vi "Main.vi"() -> ()   [LabVIEW 2024]
uses:
  1. CTL/Brain_Loop_CTL.ctl
  <vilib>/Utility/miscctls.llb/LVPointTypeDef.ctl
  <vilib>/Utility/sysdir.llb/System Directory Type.ctl
panel:
  out "Water_Velocity 10":dbl
  out "Water_Velocity 9":dbl
  out "Water_Velocity 8":dbl
  out "Water_Velocity 7":dbl
  out "Water_Velocity 6":dbl
  out "Water_Velocity 5":dbl
  out "Water_Velocity 4":dbl
  out "Water_Velocity 3":dbl
  out "Water_Velocity 2":dbl
  out "Water_Velocity":dbl
  in  "숫자형":i32
  in  "유속 데이터 흐름표_50분":i32(listbox)=-1
  in  "유속 데이터 흐름표_30분":i32(listbox)=-1
  in  "유속 데이터 흐름표_10분":i32(listbox)=-1
  in  "유속 데이터":T1
  in  "데이터 통계":T2
  in  "관리자":T3
  out "반환값":string
  in  "전체메뉴_탭_컨트롤":enum32{"지도", "데이터 통계", "관리자", "유속 데이터"}(tab)=enum."데이터 통계"
  out "Station_5_수신시작시간":string
  out "Station_4_수신시작시간":string
  out "Station_3_수신시작시간":string
  out "Station_2_수신시작시간":string
  out "Station_1_수신시작시간":string
  out "Station_5":cluster{dbl[], i32[]}(graph)
  out "TX_LED_5":bool
  out "RX_LED_5":bool
  out "Station_4":cluster{dbl[], i32[]}(graph)
  out "TX_LED_4":bool
  out "RX_LED_4":bool
  out "Station_3":cluster{dbl[], i32[]}(graph)
  out "TX_LED_3":bool
  out "RX_LED_3":bool
  out "Station_2":cluster{dbl[], i32[]}(graph)
  out "TX_LED_2":bool
  out "RX_LED_2":bool
  out "Station_1":cluster{dbl[], i32[]}(graph)
  out "TX_LED_1":bool
  out "RX_LED_1":bool
  in  "관리자_내부_탭_컨트롤":enum32{"실시간 현황", "Setting"}(tab) caption="탭 컨트롤 2"
  out "Station_현황_GPS":i32[](listbox)
  out "데이터 통계 현황_결과창":string
  out "Station_현황_TRX_Controller":i32[](listbox)
  in  "Python 경로":path=path "D:/Python39-32/python.exe"
  out "적용_LED":bool
  in  "적용 버튼":bool
  in  "정지":bool
  in  "Publish_모듈 경로":path=path "C:/Users/user/Desktop/CATS_V4.0/5. Python/Mqtt_Publish_Client.py"
  in  "Subscribe_모듈 경로":path=path "C:/Users/user/Desktop/CATS_V4.0/5. Python/Mqtt_Subscribe_Client.py"
  in  "지도 모듈 경로":path=path "C:/Users/user/Desktop/CATS_V4.0/5. Python/Generate_map.py"
  out "적용_LED 2":bool
  in  "Wake_UP버튼":bool
  out "지도모듈_LED":bool
  in  "지도":T4
  in  "Order":i32=12
  in  "Q 값":i32=4
  # "Costal Acoustic Tomography(Ver1.1)"
  # "데이터 통계 현황"
  # "Costal Acoustic Tomography Setting"
  # "Data_path"
  # "Coastal_TMC_Set_Variable"
  # "Coastal_TMC_Map_Web"
  # "Sation_Wake_UP"
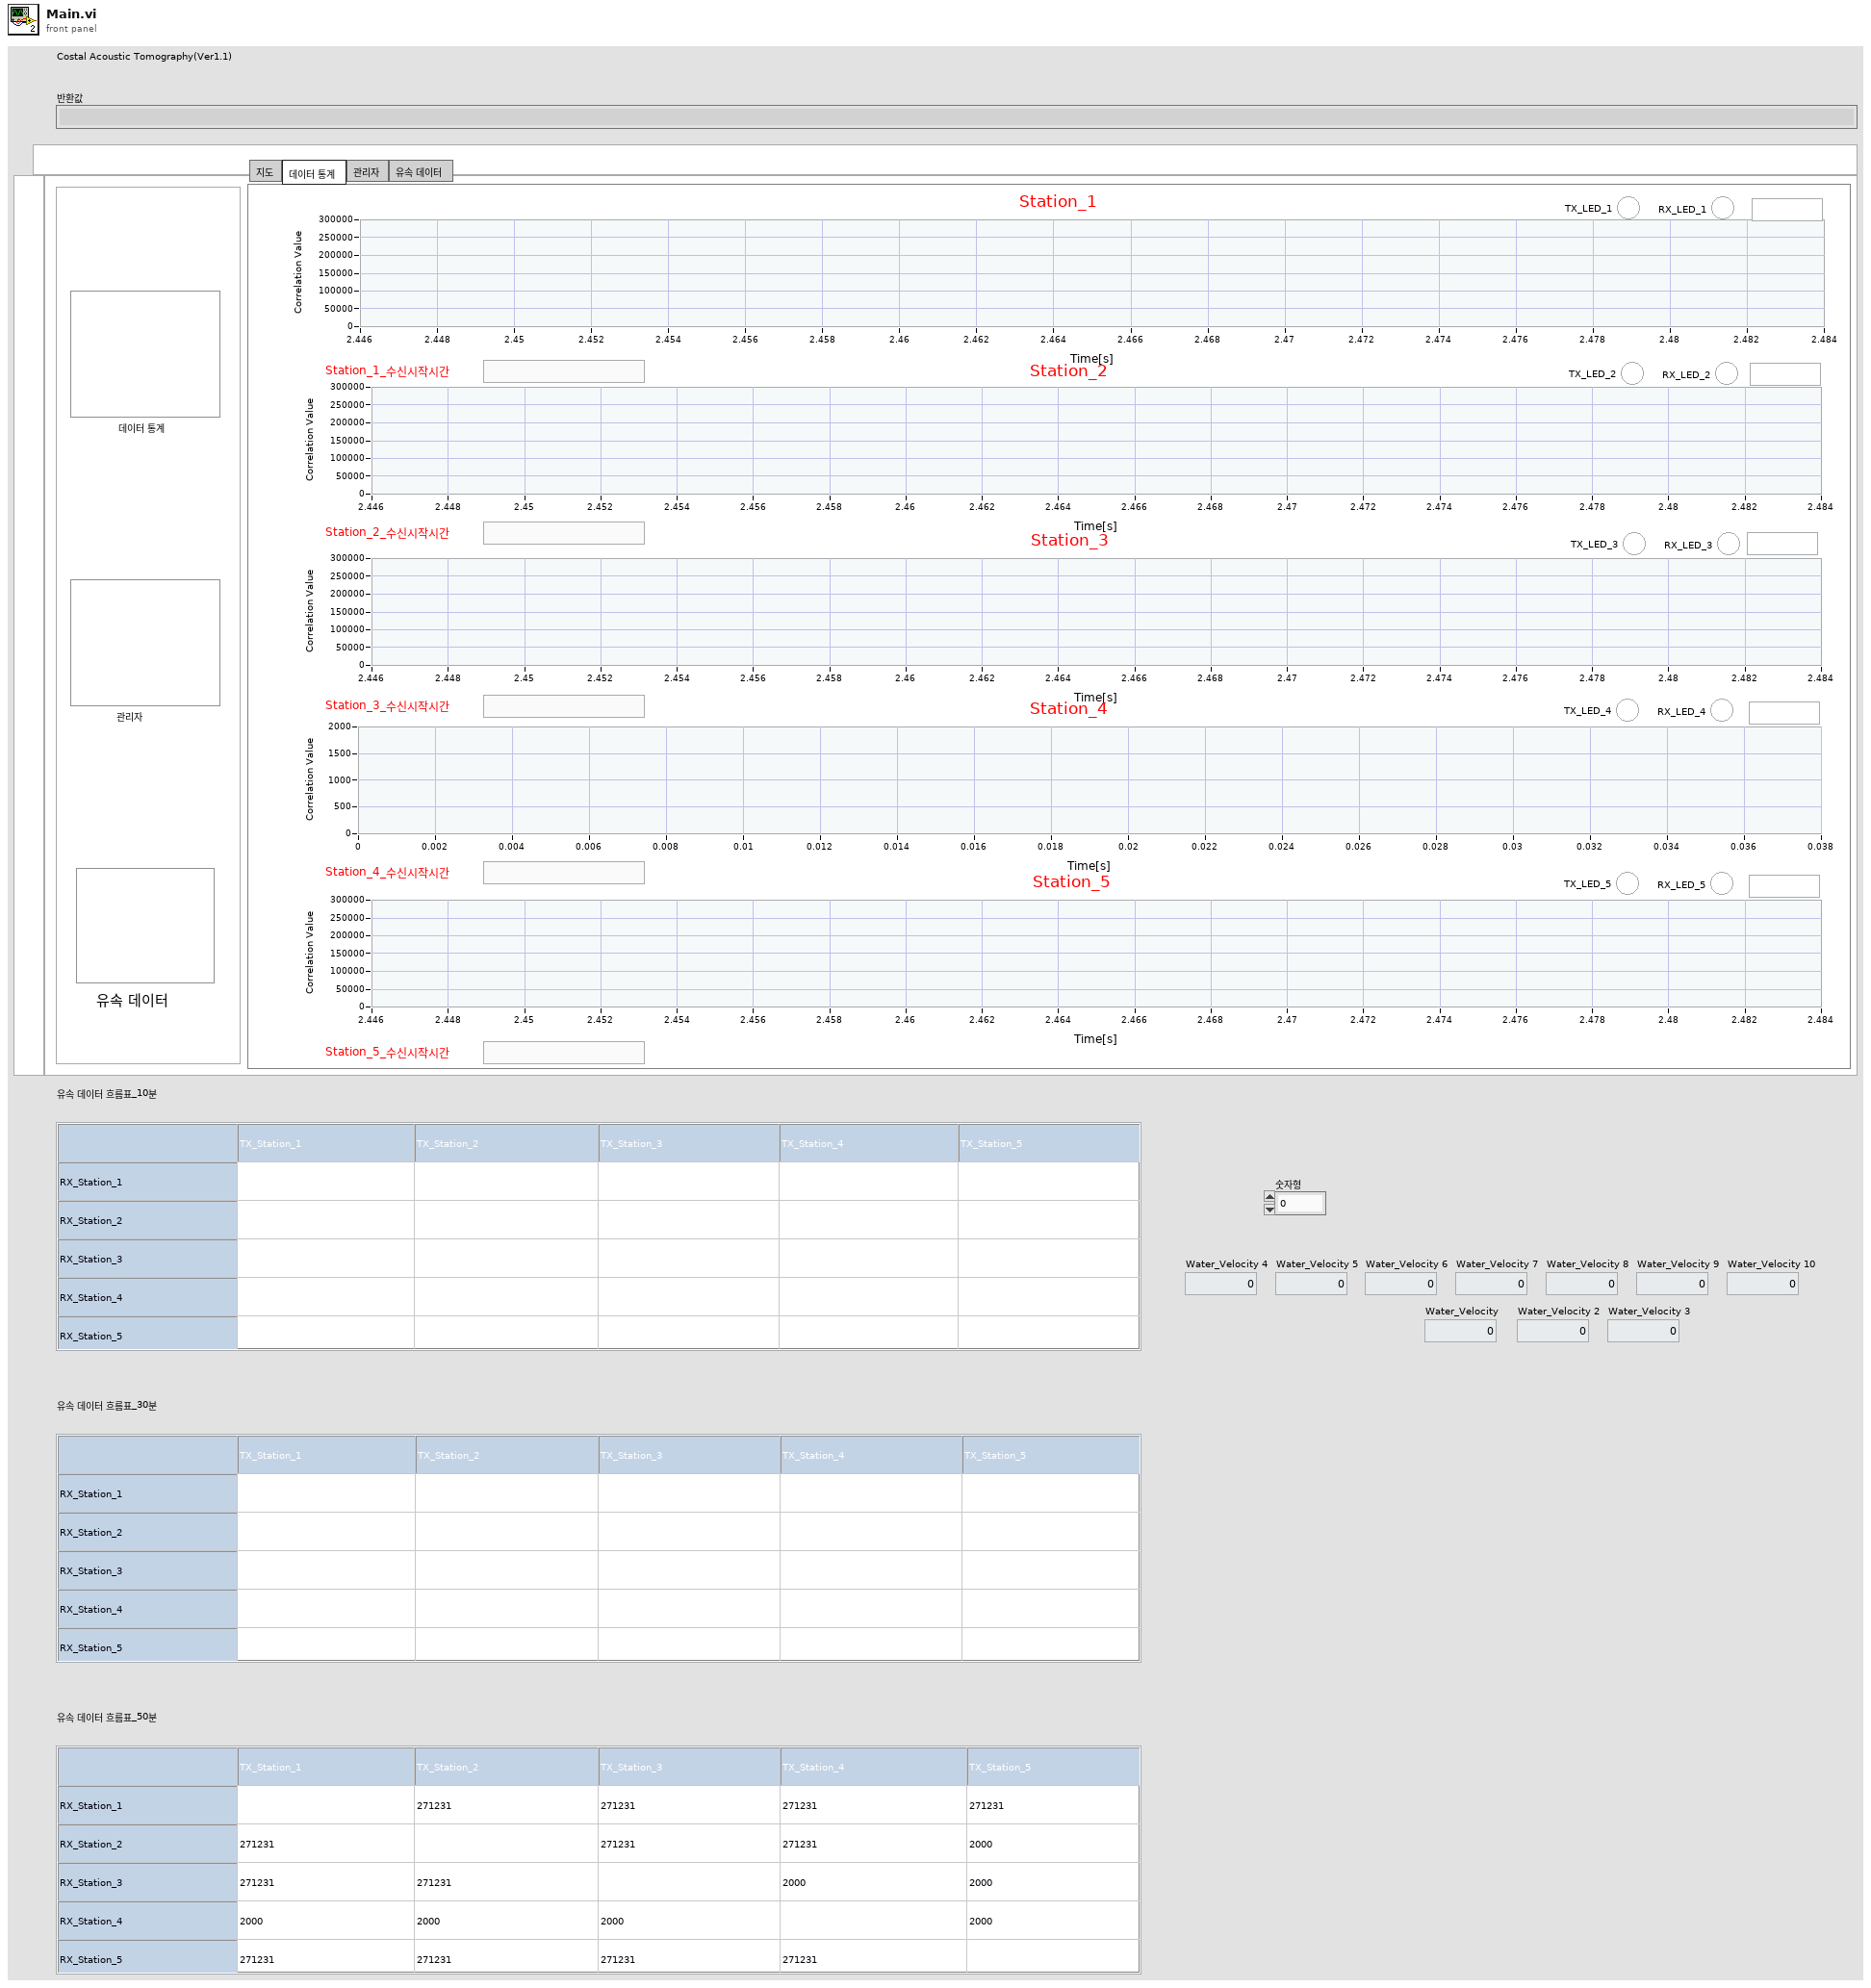
[diagram p1: front panel]
types:
  T1 = typedef "알림 컨트롤.ctl" = bool
  T2 = typedef "데이터 컨트롤.ctl" = bool
  T3 = typedef "관리 컨트롤.ctl" = bool
  T4 = typedef "지도 컨트롤.ctl" = bool
  T5 = cluster{"로그기록":string, "RX_그래프_LED":bool, "RX_그래프2_LED":bool, "RX_그래프3_LED":bool, "RX_그래프4_LED":bool, "RX_그래프5_LED":bool}
  T6 = cluster{"TX_그래프_LED":bool, "TX_그래프2_LED":bool, "TX_그래프3_LED":bool, "TX_그래프4_LED":bool, "TX_그래프5_LED":bool, "유속데이터흐름표_10분":string[][], "유속데이터흐름표_30분":string[][], "유속데이터흐름표_50분":string[][]}
  T7 = cluster{"Python 경로":path, "Publish 모듈 경로":path, "지도 모듈 경로":path}
  T8 = cluster{"TX_그래프_LED":bool, "TX_그래프2_LED":bool, "TX_그래프3_LED":bool, "TX_그래프4_LED":bool, "TX_그래프5_LED":bool}
  T9 = typedef "Brain_Loop_CTL.ctl" = enum16{"초기화", "Mqtt_Subscribe", "Mqtt_Publish", "지도", "관리자", "데이터통계", "유속 데이터", "정지", "Mqtt_Publish_2"}
  T10 = typedef "LVPointTypeDef.ctl" = cluster{"Horizontal":i16, "Vertical":i16}
  T11 = typedef "System Directory Type.ctl" = i32
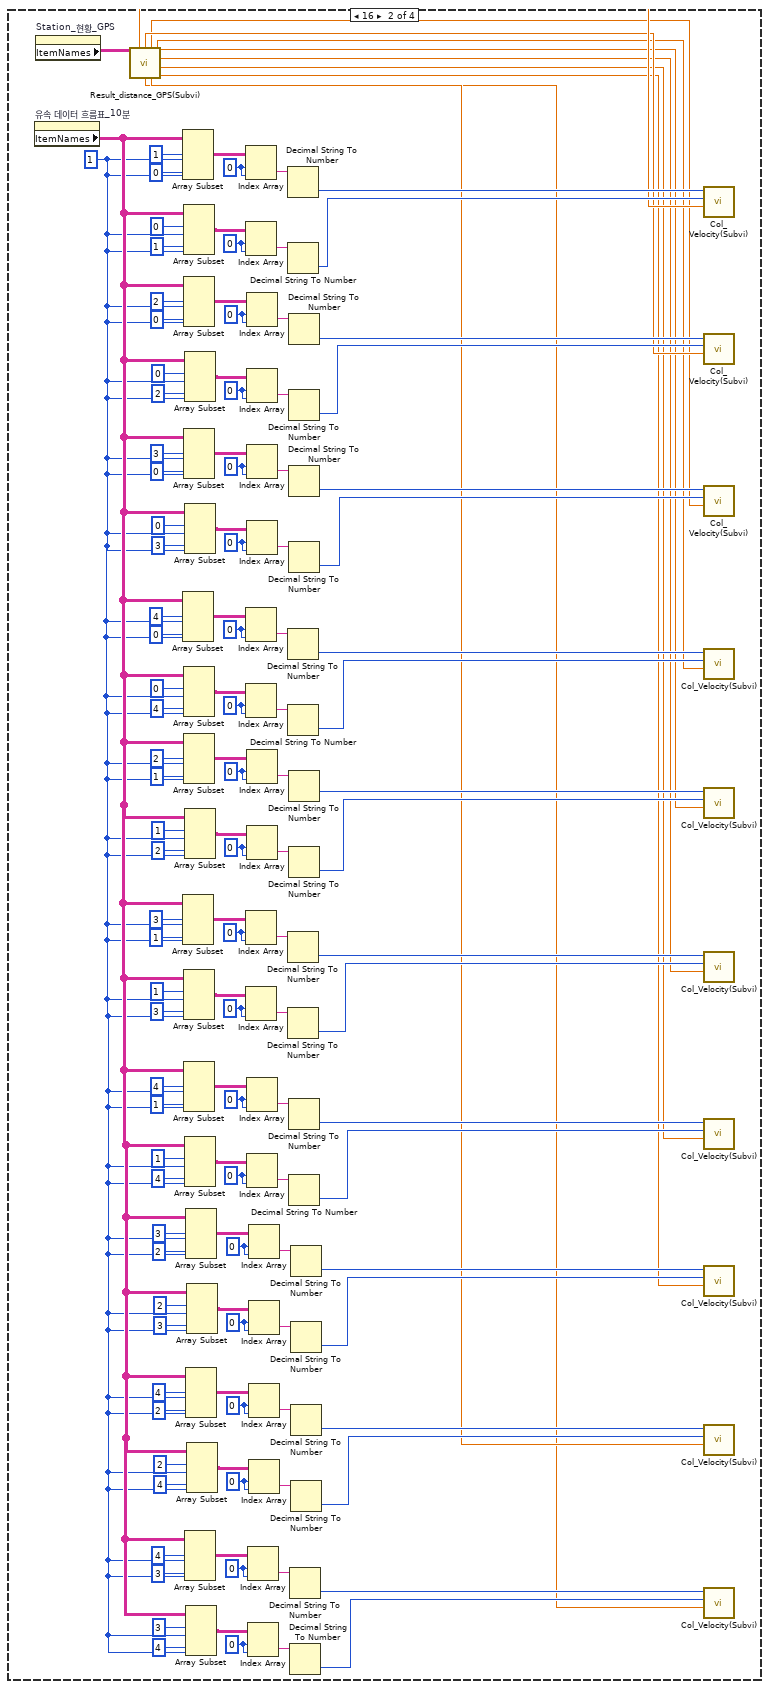
[diagram p3: hidden frame]
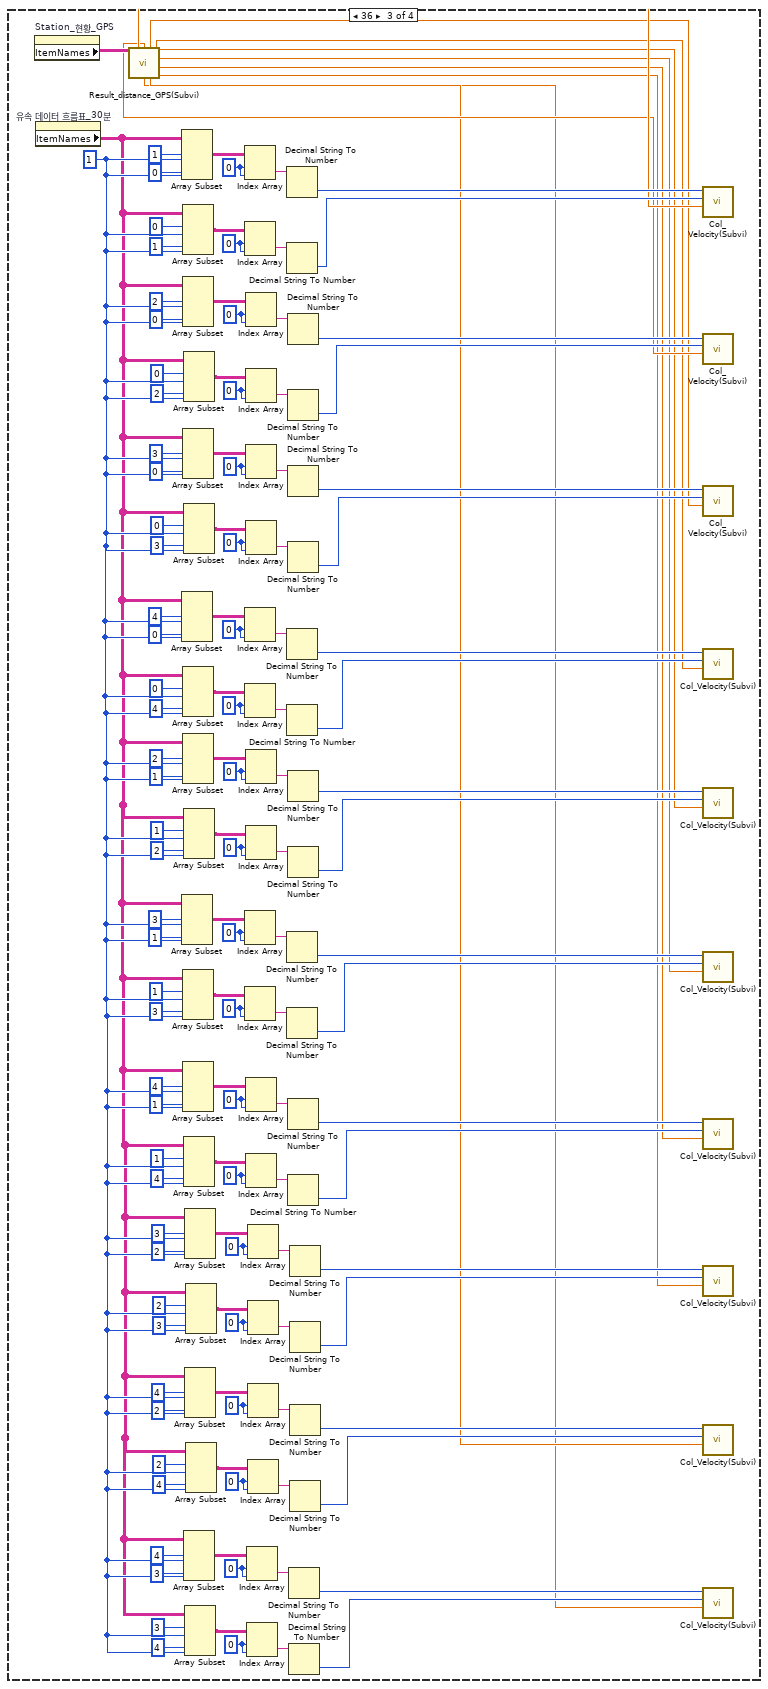
[diagram p4: hidden frame]
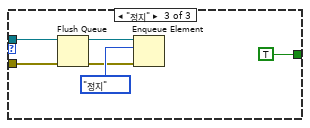
[diagram p6: hidden frame]
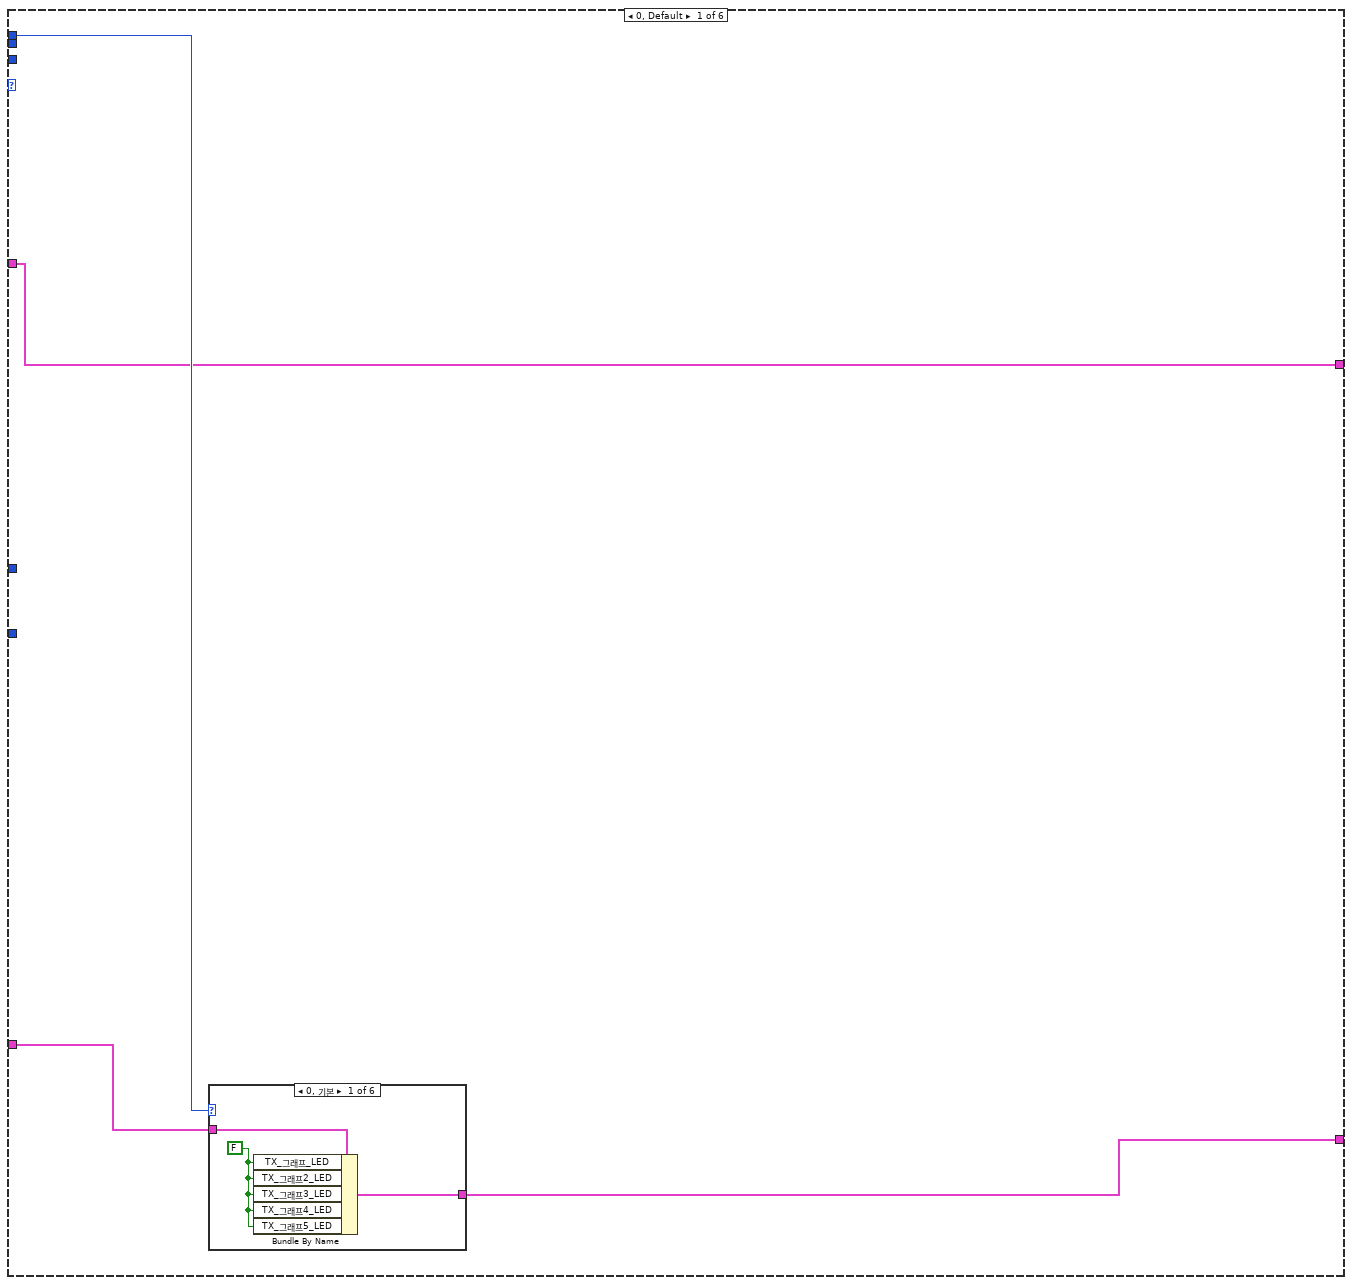
[diagram p7: hidden frame]
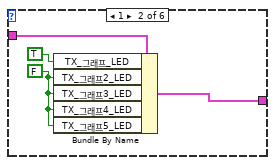
[diagram p8: hidden frame]
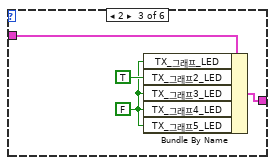
[diagram p9: hidden frame]
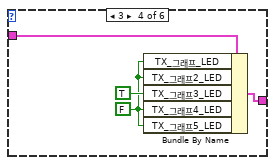
[diagram p10: hidden frame]
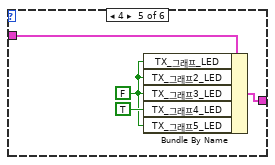
[diagram p11: hidden frame]
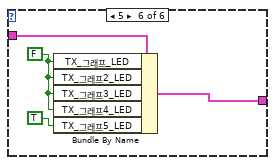
[diagram p12: hidden frame]
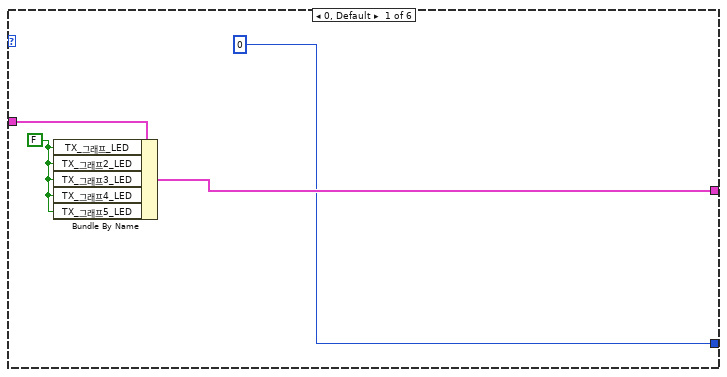
[diagram p13: hidden frame]
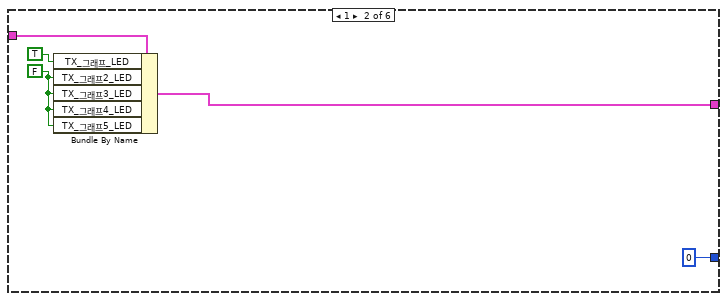
[diagram p14: hidden frame]
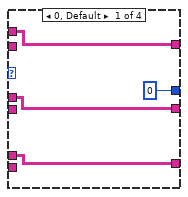
[diagram p15: hidden frame]
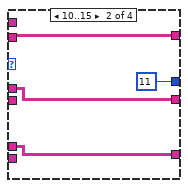
[diagram p16: hidden frame]
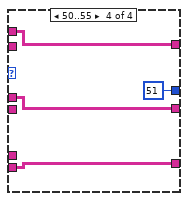
[diagram p17: hidden frame]
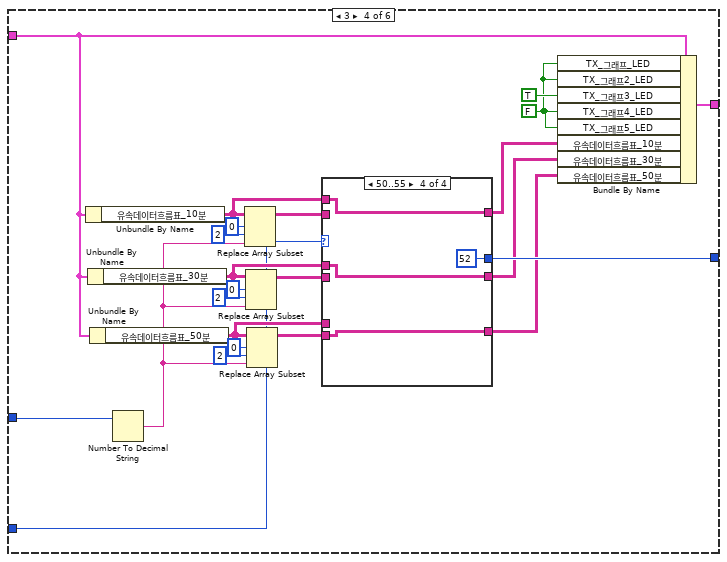
[diagram p18: hidden frame]
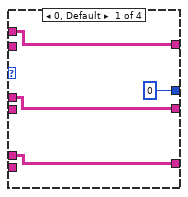
[diagram p19: hidden frame]
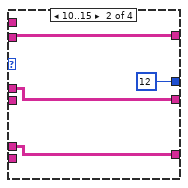
[diagram p20: hidden frame]
diagram:
  (unwired) T8 {"TX_그래프_LED"=FALSE, "TX_그래프2_LED"=FALSE, "TX_그래프3_LED"=FALSE, "TX_그래프4_LED"=FALSE, "TX_그래프5_LED"=FALSE}
  w20 = string[] []
  w21 = Brain_Loop_CTL."초기화"
  # "※ 현재 시간과 비교하여 10분 인지 30분인지 50분 출력 모듈 추가"
  # "Queue4: GPSDATA_처리 LOOP"
  # "GPS_리스트 박스 데이터 초기 값"
  # "TRX_Controller_리스트 박스 데이터 초기 값"
  # "Date: 2024.02.05\nTitle: Costal Acoustic Tmography GUI V1.1\nBy: KangJinSeong"
  n1 = Obtain Queue(element data type=w20) -> (queue out=w19:refnum<queue>, error out=w18:errorcluster)  [unwired: 4 in, 1 out]
  n2 = Obtain Queue(element data type=w20) -> (queue out=w7:refnum<queue>, error out=w6:errorcluster)  [unwired: 4 in, 1 out]
  n3 = Obtain Queue(element data type=w20) -> (queue out=w17:refnum<queue>, error out=w16:errorcluster)  [unwired: 4 in, 1 out]
  n4 = Obtain Queue(element data type=w21) -> (queue out=w24:refnum<queue>, error out=w26:errorcluster)  [unwired: 4 in, 1 out]
  n5 = Obtain Queue(element data type=w21) -> (queue out=w2:refnum<queue>, error out=w1:errorcluster)  [unwired: 4 in, 1 out]
  n6 = Enqueue Element(queue=w24, element=w21, error in (no error)=w26) -> (queue out=w15:refnum<queue>, error out=w25:errorcluster)  [unwired: 1 in, 1 out]
  n7 = while {
    tunnel: w15 -> [w29]
    shift-right: [w28] -> w23
    shift-left: w25 -> [w30]
    stop <- w27 stop-if-true
    n8 = event shown="[6] \"정지\": 값 변경" {
      selector: _ -> [_ _ _ _ _ _ _]
      dyn-events: _ -> [_ _ _ _ _ _ _]
      timeout: _ -> [_ _ _ _ _ _ _]
      tunnel: w30 -> [w35 w40 w42 w47 w55 w60 w66]
      tunnel: w29 -> [w34 w39 w44 w49 w54 w59 w65]
      tunnel: [w32 w37 w43 w48 w52 w58 w63] -> _
      tunnel: [w31 w36 w41 w46 w51 w57 w62] -> w28
      tunnel: [_ _ _ _ _ _ TRUE] -> w27
      event Value Change {
        n9 = event-data() -> ()  [unwired: 1 in, 1 out]
        n10 = Enqueue Element(queue=w34, element=Brain_Loop_CTL."지도", error in (no error)=w35) -> (queue out=w32:refnum<queue>, error out=w31:errorcluster)  [unwired: 1 in, 1 out]
      }
      event Value Change {
        n11 = event-data() -> ()  [unwired: 1 in, 1 out]
        n12 = Enqueue Element(queue=w39, element=Brain_Loop_CTL."데이터통계", error in (no error)=w40) -> (queue out=w37:refnum<queue>, error out=w36:errorcluster)  [unwired: 1 in, 1 out]
      }
      event "적용 버튼": Value Change {
        n13 = event-data() -> ()  [unwired: 1 in, 1 out]
        n14 = Enqueue Element(queue=w44, element=Brain_Loop_CTL."Mqtt_Publish", error in (no error)=w42) -> (queue out=w43:refnum<queue>, error out=w41:errorcluster)  [unwired: 1 in, 1 out]
      }
      event "Wake_UP버튼": Value Change {
        n15 = event-data() -> ()  [unwired: 1 in, 1 out]
        n16 = Enqueue Element(queue=w49, element=Brain_Loop_CTL."Mqtt_Publish_2", error in (no error)=w47) -> (queue out=w48:refnum<queue>, error out=w46:errorcluster)  [unwired: 1 in, 1 out]
      }
      event Value Change {
        n17 = event-data() -> ()  [unwired: 1 in, 1 out]
        n18 = Enqueue Element(queue=w54, element=Brain_Loop_CTL."관리자", error in (no error)=w55) -> (queue out=w52:refnum<queue>, error out=w51:errorcluster)  [unwired: 1 in, 1 out]
      }
      event Value Change {
        n19 = event-data() -> ()  [unwired: 1 in, 1 out]
        n20 = Enqueue Element(queue=w59, element=Brain_Loop_CTL."유속 데이터", error in (no error)=w60) -> (queue out=w58:refnum<queue>, error out=w57:errorcluster)  [unwired: 1 in, 1 out]
      }
      event "정지": Value Change {
        n21 = event-data() -> ()  [unwired: 1 in, 1 out]
        n22 = Enqueue Element(queue=w65, element=Brain_Loop_CTL."정지", error in (no error)=w66) -> (queue out=w63:refnum<queue>, error out=w62:errorcluster)  [unwired: 1 in, 1 out]
      }
    }
  }
  n23 = while {
    tunnel: w2 -> [w79]
    tunnel: w1 -> [w78]
    tunnel: w19 -> [w74]
    tunnel: w18 -> [w73]
    tunnel: [errorcluster {"status"=FALSE, "code"=0, "source"=""} ("에러 상수")] -> w12
    tunnel: w7 -> [w71]
    tunnel: w6 -> [w70]
    tunnel: w17 -> [w69]
    tunnel: w16 -> [w68]
    stop <- w77 stop-if-true
    # "Mqtt_Subscribe_Loop\n※ Brain_Loop의 Queue 값의 따라 작동(Mqtt_Subscribe, 정지, 초기화)"
    n24 = Dequeue Element(queue=w79, error in (no error)=w78) -> (queue out=w76:refnum<queue>, element=w67:T9, error out=w75:errorcluster)  [unwired: 1 in, 1 out]
    n25 = case shown="\"Mqtt_Subscribe\"" w67 {
      tunnel: [_ _ TRUE] -> w77
      tunnel: w76 -> [_ w100 w108]
      tunnel: w75 -> [_ w99 w107]
      tunnel: w74 -> [_ w97 _]
      tunnel: w73 -> [_ w96 _]
      tunnel: w71 -> [_ w95 _]
      tunnel: w70 -> [_ w94 _]
      tunnel: w69 -> [_ w93 _]
      tunnel: w68 -> [_ w92 _]
      frame "초기화", Default {
      }
      frame "Mqtt_Subscribe" {
        # "※ Queue 값의 따라 Python 모듈을 실행 해당 값을 통해 각 Loop 값에 데이터 전달"
        n26 = local read "Python 경로"() -> (w80:path)
        n27 = Enqueue Element(queue=w100, element=Brain_Loop_CTL."Mqtt_Subscribe", error in (no error)=w99) -> ()  [unwired: 1 in, 3 out]
        n28 = Open Python Session(python version="3.9" ("Python 버전"), python path=w80) -> (session out=w86:refnum<k35>, error out=w102:errorcluster)  [unwired: 1 in]
        n29 = node(w86, "Subscribe_모듈 경로", "Mqtt_Subscribe" ("함수 이름"), w102, "") -> (w88:refnum<k35>, w87:errorcluster, w83:string)  [unwired: 2 out]
        "반환값" <- w83
        n30 = Close Python Session(session in=w88, error in=w87) -> (11:w82:errorcluster)
        n31 = call "Split_Queue(Subvi).vi"("입력 문자열"=w83) -> ("Split_Queue2_Result"=w91:string[], "Split_Queue3_Result"=w90:string[], "Split_Queue4_Result"=w89:string[])  [unwired: 5 in, 3 out]
        n32 = call <vilib>:"Clear Errors.vi"("error in (no error)"=w82, "specific error code to clear (0: all)"=0) -> ()  [unwired: 4 in, 2 out]
        n33 = Enqueue Element(queue=w97, element=w91, error in (no error)=w96) -> ()  [unwired: 1 in, 3 out]
        n34 = Enqueue Element(queue=w93, element=w89, error in (no error)=w92) -> ()  [unwired: 1 in, 3 out]
        n35 = Enqueue Element(queue=w95, element=w90, error in (no error)=w94) -> ()  [unwired: 1 in, 3 out]
      }
      frame "정지" {
        # "※ Queue 값의 따라 정지 인경우 해당 큐를 비우고 정지 전달"
        n36 = Flush Queue(queue=w108, error in (no error)=w107) -> (queue out=w106:refnum<queue>, error out=w105:errorcluster)  [unwired: 1 out]
        n37 = Enqueue Element(queue=w106, element=Brain_Loop_CTL."정지", error in (no error)=w105) -> ()  [unwired: 1 in, 3 out]
      }
    }
  }
  n38 = while "While 루프" {
    tunnel: w2 -> [w144]
    tunnel: w1 -> [w143]
    tunnel: w7 -> [w142]
    tunnel: w6 -> [w141]
    shift-right: [w124] -> _
    shift-left: T6 {"TX_그래프_LED"=FALSE, "TX_그래프2_LED"=FALSE, "TX_그래프3_LED"=FALSE, "TX_그래프4_LED"=FALSE, "TX_그래프5_LED"=FALSE, "유속데이터흐름표_10분"=[["", "", "", "", "", ""], ["", "", "", "", "", ""], ["", "", "", "", "", ""], ["", "", "", "", "", ""], ["", "", "", "", "", ""], ["", "", "", "", "", "0"]], "유속데이터흐름표_30분"=[["", "", "", "", "", ""], ["", "", "", "", "", ""], ["", "", "", "", "", ""], ["", "", "", "", "", ""], ["", "", "", "", "", ""], ["", "", "", "", "", "0"]], "유속데이터흐름표_50분"=[["", "", "", "", "", ""], ["", "", "", "", "", ""], ["", "", "", "", "", ""], ["", "", "", "", "", ""], ["", "", "", "", "", ""], ["", "", "", "", "", "0"]]} -> [w130]
    shift-right: [w119] -> _
    shift-left: T5 {"로그기록"="", "RX_그래프_LED"=FALSE, "RX_그래프2_LED"=FALSE, "RX_그래프3_LED"=FALSE, "RX_그래프4_LED"=FALSE, "RX_그래프5_LED"=FALSE} -> [w123]
    stop <- w145 stop-if-true
    # "※ Queue3 처리 LOOP에 데이터가 들어오는 경우 각 인덱스에 맞게 데이터 분리 후 웨이브폼 그래프에 표시\n   TX_Station/RX_Station 값에 따라 .CSV 파일로 데이터 저장"
    # "※ TX_Station 번호 별로 그래프 하단에 LED 점멸(빨간색)\n    RX_Station 번호 별로 그래프 하단에 LED 점멸(파란색)"
    # "0 index: TX_Station\n1 index: RX_Station\n2 index: Max index"
    # "FPGA 신호처리된 결과값"
    # "Queue3: SIGDATA 처리 LOOP\n신호처리된 데이터 가시화 경우 시간 데이터로 표시"
    n39 = Dequeue Element(queue=w144, error in (no error)=w143) -> (queue out=w147:refnum<queue>, element=w146:T9, error out=w148:errorcluster)  [unwired: 1 in, 1 out]
    n40 = Dequeue Element(queue=w142, error in (no error)=w141) -> (element=w140:string[])  [unwired: 1 in, 3 out]
    n41 = case shown="\"Mqtt_Subscribe\"" w146 {
      tunnel: [_ _ TRUE] -> w145
      tunnel: w147 -> [_ w1327 w1332]
      tunnel: w148 -> [_ w1326 w1331]
      frame "초기화", Default {
      }
      frame "Mqtt_Subscribe" {
        n42 = Enqueue Element(queue=w1327, element=Brain_Loop_CTL."Mqtt_Subscribe", error in (no error)=w1326) -> ()  [unwired: 1 in, 3 out]
      }
      frame "정지" {
        n43 = Flush Queue(queue=w1332, error in (no error)=w1331) -> (queue out=w1330:refnum<queue>, error out=w1329:errorcluster)  [unwired: 1 out]
        n44 = Enqueue Element(queue=w1330, element=Brain_Loop_CTL."정지", error in (no error)=w1329) -> ()  [unwired: 1 in, 3 out]
      }
    }
    n45 = Decimal String To Number(string=w140) -> (number=w132:i32[])  [unwired: 2 in, 1 out]
    n46 = Array Subset(array=w132, index=4 ("인덱스"), length=4000 ("길이")) -> ()  [unwired: 1 out]
    n47 = Index Array(array=w132, index #1=1 ("인덱스"), index #2=0 ("인덱스"), index #3=2 ("인덱스")) -> (element #1=w133:i32, element #2=w134:i32, element #3=w131:i32)
    n48 = local read "Order"() -> (w121:i32)
    n49 = local read "Q 값"() -> (w122:i32)
    n50 = case shown="1" w133 {
      tunnel: w134 -> [w152 w209 w414 w642 w870 w1100]
      tunnel: w133 -> [_ w208 w435 w669 w898 w1128]
      tunnel: w132 -> [_ w225 w455 w685 w915 w1145]
      tunnel: w131 -> [_ w179 w411 w641 w869 w1099]
      tunnel: w130 -> [w151 w223 w413 w643 w871 w1101]
      tunnel: [w150 w222 w410 w639 w872 w1102] -> w124
      tunnel: w123 -> [w149 w205 w436 w670 w899 w1129]
      tunnel: w122 -> [_ w207 w438 w668 w897 w1127]
      tunnel: w121 -> [_ w206 w437 w667 w896 w1126]
      tunnel: [w149 w201 w439 w671 w900 w1130] -> w119
      tunnel: 50 -> [_ w176 w406 w636 w866 w1096]
      frame 0, Default {
        n51 = case shown="0, 기본" w152 {
          tunnel: w151 -> [w155 w159 w163 w167 w171 w175]
          tunnel: [w154 w156 w162 w166 w170 w174] -> w150
          frame 0, Default {
            w153 = FALSE
            n52 = Bundle By Name(cluster=w155, "TX_그래프_LED"=w153, "TX_그래프2_LED"=w153, "TX_그래프3_LED"=w153, "TX_그래프4_LED"=w153, "TX_그래프5_LED"=w153) -> (w154:T6)
          }
          frame 1 {
            w157 = FALSE
            n53 = Bundle By Name(cluster=w159, "TX_그래프_LED"=TRUE, "TX_그래프2_LED"=w157, "TX_그래프3_LED"=w157, "TX_그래프4_LED"=w157, "TX_그래프5_LED"=w157) -> (w156:T6)
          }
          frame 2 {
            w160 = FALSE
            n54 = Bundle By Name(cluster=w163, "TX_그래프_LED"=w160, "TX_그래프2_LED"=TRUE, "TX_그래프3_LED"=w160, "TX_그래프4_LED"=w160, "TX_그래프5_LED"=w160) -> (w162:T6)
          }
          frame 3 {
            w164 = FALSE
            n55 = Bundle By Name(cluster=w167, "TX_그래프_LED"=w164, "TX_그래프2_LED"=w164, "TX_그래프3_LED"=TRUE, "TX_그래프4_LED"=w164, "TX_그래프5_LED"=w164) -> (w166:T6)
          }
          frame 4 {
            w168 = FALSE
            n56 = Bundle By Name(cluster=w171, "TX_그래프_LED"=w168, "TX_그래프2_LED"=w168, "TX_그래프3_LED"=w168, "TX_그래프4_LED"=TRUE, "TX_그래프5_LED"=w168) -> (w170:T6)
          }
          frame 5 {
            w172 = FALSE
            n57 = Bundle By Name(cluster=w175, "TX_그래프_LED"=w172, "TX_그래프2_LED"=w172, "TX_그래프3_LED"=w172, "TX_그래프4_LED"=w172, "TX_그래프5_LED"=TRUE) -> (w174:T6)
          }
        }
      }
      frame 1 {
        w202 = FALSE
        # "※ 현재 시간과 비교하여 10분 인지 30분인지 50분 출력 모듈 추가"
        # "※2차원 벡터 -> 1차원 벡터"
        n58 = Subtract(x=w179, y=2000) -> (x-y=w228:i32)
        n59 = Format Date/Time String(time format string (%c)="%M" ("시간 포맷 문자열 (%c)")) -> (date/time string=w178:string)  [unwired: 2 in]
        n60 = call "Save_Log_File(Subvi).vi"("TX_Station"=w209, "RX_Station"=w208, "1D data"=w225) -> ()  [unwired: 7 in, 1 out]
        n61 = property on="Station_현황_TRX_Controller" class="MCListbox (엄격한)"() -> ("ItemNames"=w196:string[][])  [unwired: 2 in, 2 out]
        n62 = for {
          N: 4001 -> [_]
          tunnel: w228 -> [w405]
          shift-right: [w400] -> w226
          shift-left: dbl[] [] -> [w402]
          i -> [w399]
          n63 = Add(x=w405, y=w399) -> (x+y=w404:i32)
          n64 = Divide(x=w404, y=110000) -> (x/y=w401:dbl)
          n65 = Build Array (concatenate)(w402, w401) -> (w400:dbl[])
        }
        n66 = Unbundle By Name(w205) -> ("로그기록"=w210:string)
        n67 = Number To Decimal String(number=w209) -> (decimal integer string=w189:string)  [unwired: 1 in]
        n68 = Number To Decimal String(number=w208) -> (decimal integer string=w188:string)  [unwired: 1 in]
        n69 = Number To Decimal String(number=w179) -> (decimal integer string=w187:string)  [unwired: 1 in]
        n70 = Number To Decimal String(number=w207) -> (decimal integer string=w217:string)  [unwired: 1 in]
        n71 = Number To Decimal String(number=w206) -> (decimal integer string=w216:string)  [unwired: 1 in]
        n72 = Decimal String To Number(string=w178) -> ()  [unwired: 2 in, 2 out]
        n73 = Concatenate Strings("_Q_" ("시간 포맷 문자열 (%c)"), w217) -> (w214:string)
        n74 = Concatenate Strings("_Order : " ("시간 포맷 문자열 (%c)"), w216) -> (w213:string)
        n75 = case shown="2" w209 {
          tunnel: w223 -> [w237 w242 w256 w288 w327 w364]
          tunnel: [w236 w239 w259 w304 w343 w382] -> w222
          tunnel: [0 0 w263 w286 w325 w366] -> w199
          tunnel: w179 -> [_ _ w260 w287 w326 w365]
          tunnel: w176 -> [_ _ w243 w282 w321 w360]
          frame 0, Default {
            w235 = FALSE
            n76 = Bundle By Name(cluster=w237, "TX_그래프_LED"=w235, "TX_그래프2_LED"=w235, "TX_그래프3_LED"=w235, "TX_그래프4_LED"=w235, "TX_그래프5_LED"=w235) -> (w236:T6)
          }
          frame 1 {
            w240 = FALSE
            n77 = Bundle By Name(cluster=w242, "TX_그래프_LED"=TRUE, "TX_그래프2_LED"=w240, "TX_그래프3_LED"=w240, "TX_그래프4_LED"=w240, "TX_그래프5_LED"=w240) -> (w239:T6)
          }
          frame 2 {
            w264 = FALSE
            n78 = Unbundle By Name(w256) -> ("유속데이터흐름표_10분"=w244:string[][])
            n79 = Unbundle By Name(w256) -> ("유속데이터흐름표_30분"=w246:string[][])
            n80 = Unbundle By Name(w256) -> ("유속데이터흐름표_50분"=w245:string[][])
            n81 = Number To Decimal String(number=w260) -> (decimal integer string=w253:string)  [unwired: 1 in]
            n82 = Replace Array Subset(array=w244, new element=w253, index (row)=0 ("인덱스 (행)"), index (col)=1 ("비활성화된 인덱스 (열)")) -> (w252:string[][])
            n83 = Replace Array Subset(array=w246, new element=w253, index (row)=0 ("인덱스 (행)"), index (col)=1 ("비활성화된 인덱스 (열)")) -> (w251:string[][])
            n84 = Replace Array Subset(array=w245, new element=w253, index (row)=0 ("인덱스 (행)"), index (col)=1 ("비활성화된 인덱스 (열)")) -> (w250:string[][])
            n85 = case shown="30..35" w243 {
              tunnel: [0 11 31 51] -> w263
              tunnel: w252 -> [_ w272 _ _]
              tunnel: w251 -> [_ _ w275 _]
              tunnel: w250 -> [_ _ _ w278]
              tunnel: [w268 w272 w276 w280] -> w249
              tunnel: [w267 w271 w275 w279] -> w248
              tunnel: [w266 w270 w274 w278] -> w247
              tunnel: w246 -> [w267 w271 _ w279]
              tunnel: w245 -> [w266 w270 w274 _]
              tunnel: w244 -> [w268 _ w276 w280]
              frame 0, Default {
              }
              frame 10..15 {
              }
              frame 30..35 {
              }
              frame 50..55 {
              }
            }
            n86 = Bundle By Name(cluster=w256, "TX_그래프_LED"=w264, "TX_그래프2_LED"=TRUE, "TX_그래프3_LED"=w264, "TX_그래프4_LED"=w264, "TX_그래프5_LED"=w264, "유속데이터흐름표_10분"=w249, "유속데이터흐름표_30분"=w248, "유속데이터흐름표_50분"=w247) -> (w259:T6)
          }
          frame 3 {
            w302 = FALSE
            n87 = Unbundle By Name(w288) -> ("유속데이터흐름표_10분"=w301:string[][])
            n88 = Unbundle By Name(w288) -> ("유속데이터흐름표_30분"=w299:string[][])
            n89 = Unbundle By Name(w288) -> ("유속데이터흐름표_50분"=w300:string[][])
            n90 = Number To Decimal String(number=w287) -> (decimal integer string=w295:string)  [unwired: 1 in]
            n91 = Replace Array Subset(array=w301, new element=w295, index (row)=0 ("인덱스 (행)"), index (col)=2 ("비활성화된 인덱스 (열)")) -> (w296:string[][])
            n92 = Replace Array Subset(array=w299, new element=w295, index (row)=0 ("인덱스 (행)"), index (col)=2 ("비활성화된 인덱스 (열)")) -> (w297:string[][])
            n93 = Replace Array Subset(array=w300, new element=w295, index (row)=0 ("인덱스 (행)"), index (col)=2 ("비활성화된 인덱스 (열)")) -> (w298:string[][])
            n94 = case shown="50..55" w282 {
              tunnel: [0 12 32 52] -> w286
              tunnel: w296 -> [_ w311 _ _]
              tunnel: w297 -> [_ _ w314 _]
              tunnel: w298 -> [_ _ _ w317]
              tunnel: [w307 w311 w315 w319] -> w285
              tunnel: [w306 w310 w314 w318] -> w284
              tunnel: [w305 w309 w313 w317] -> w283
              tunnel: w299 -> [w306 w310 _ w318]
              tunnel: w300 -> [w305 w309 w313 _]
              tunnel: w301 -> [w307 _ w315 w319]
              frame 0, Default {
              }
              frame 10..15 {
              }
              frame 30..35 {
              }
              frame 50..55 {
              }
            }
            n95 = Bundle By Name(cluster=w288, "TX_그래프_LED"=w302, "TX_그래프2_LED"=w302, "TX_그래프3_LED"=TRUE, "TX_그래프4_LED"=w302, "TX_그래프5_LED"=w302, "유속데이터흐름표_10분"=w285, "유속데이터흐름표_30분"=w284, "유속데이터흐름표_50분"=w283) -> (w304:T6)
          }
          frame 4 {
            w341 = FALSE
            n96 = Unbundle By Name(w327) -> ("유속데이터흐름표_10분"=w340:string[][])
            n97 = Unbundle By Name(w327) -> ("유속데이터흐름표_30분"=w338:string[][])
            n98 = Unbundle By Name(w327) -> ("유속데이터흐름표_50분"=w339:string[][])
            n99 = Number To Decimal String(number=w326) -> (decimal integer string=w334:string)  [unwired: 1 in]
            n100 = Replace Array Subset(array=w340, new element=w334, index (row)=0 ("인덱스 (행)"), index (col)=3 ("비활성화된 인덱스 (열)")) -> (w335:string[][])
            n101 = Replace Array Subset(array=w338, new element=w334, index (row)=0 ("인덱스 (행)"), index (col)=3 ("비활성화된 인덱스 (열)")) -> (w336:string[][])
            n102 = Replace Array Subset(array=w339, new element=w334, index (row)=0 ("인덱스 (행)"), index (col)=3 ("비활성화된 인덱스 (열)")) -> (w337:string[][])
            n103 = case shown="10..15" w321 {
              tunnel: [0 13 33 53] -> w325
              tunnel: w335 -> [_ w350 _ _]
              tunnel: w336 -> [_ _ w353 _]
              tunnel: w337 -> [_ _ _ w356]
              tunnel: [w346 w350 w354 w358] -> w324
              tunnel: [w345 w349 w353 w357] -> w323
              tunnel: [w344 w348 w352 w356] -> w322
              tunnel: w338 -> [w345 w349 _ w357]
              tunnel: w339 -> [w344 w348 w352 _]
              tunnel: w340 -> [w346 _ w354 w358]
              frame 0, Default {
              }
              frame 10..15 {
              }
              frame 30..35 {
              }
              frame 50..55 {
              }
            }
            n104 = Bundle By Name(cluster=w327, "TX_그래프_LED"=w341, "TX_그래프2_LED"=w341, "TX_그래프3_LED"=w341, "TX_그래프4_LED"=TRUE, "TX_그래프5_LED"=w341, "유속데이터흐름표_10분"=w324, "유속데이터흐름표_30분"=w323, "유속데이터흐름표_50분"=w322) -> (w343:T6)
          }
          frame 5 {
            w380 = FALSE
            n105 = Unbundle By Name(w364) -> ("유속데이터흐름표_10분"=w379:string[][])
            n106 = Unbundle By Name(w364) -> ("유속데이터흐름표_30분"=w377:string[][])
            n107 = Unbundle By Name(w364) -> ("유속데이터흐름표_50분"=w378:string[][])
            n108 = Number To Decimal String(number=w365) -> (decimal integer string=w373:string)  [unwired: 1 in]
            n109 = Replace Array Subset(array=w379, new element=w373, index (row)=0 ("인덱스 (행)"), index (col)=4 ("비활성화된 인덱스 (열)")) -> (w374:string[][])
            n110 = Replace Array Subset(array=w377, new element=w373, index (row)=0 ("인덱스 (행)"), index (col)=4 ("비활성화된 인덱스 (열)")) -> (w375:string[][])
            n111 = Replace Array Subset(array=w378, new element=w373, index (row)=0 ("인덱스 (행)"), index (col)=4 ("비활성화된 인덱스 (열)")) -> (w376:string[][])
            n112 = case shown="50..55" w360 {
              tunnel: [0 14 34 54] -> w366
              tunnel: w374 -> [_ w389 _ _]
              tunnel: w375 -> [_ _ w392 _]
              tunnel: w376 -> [_ _ _ w395]
              tunnel: [w385 w389 w393 w397] -> w363
              tunnel: [w384 w388 w392 w396] -> w362
              tunnel: [w383 w387 w391 w395] -> w361
              tunnel: w377 -> [w384 w388 _ w396]
              tunnel: w378 -> [w383 w387 w391 _]
              tunnel: w379 -> [w385 _ w393 w397]
              frame 0, Default {
              }
              frame 10..15 {
              }
              frame 30..35 {
              }
              frame 50..55 {
              }
            }
            n113 = Bundle By Name(cluster=w364, "TX_그래프_LED"=w380, "TX_그래프2_LED"=w380, "TX_그래프3_LED"=w380, "TX_그래프4_LED"=w380, "TX_그래프5_LED"=TRUE, "유속데이터흐름표_10분"=w363, "유속데이터흐름표_30분"=w362, "유속데이터흐름표_50분"=w361) -> (w382:T6)
          }
        }
        n114 = Array Subset(array=w196, index (row)=0 ("인덱스"), length (row)=7 ("길이"), index (col)=0 ("인덱스"), length (col)=1 ("길이")) -> (w195:string[][])
        n115 = Format Date/Time String(time format string (%c)="%Y_%m_%d_%H_%M_" ("시간 포맷 문자열 (%c)")) -> (date/time string=w211:string)  [unwired: 2 in]
        n116 = Array Subset(array=w195, index (row)=3 ("인덱스"), length (row)=2 ("길이")) -> (w186:string[][])  [unwired: 2 in]
        n117 = Bundle(w226, w225) -> (→"Station_1":cluster{dbl[], i32[]})  [unwired: 1 in]
        n118 = for {
          tunnel: w186 -> [w232] mode=indexing
          shift-right: [w231] -> w184
          shift-left: string[] [] -> [w233]
          n119 = Build Array (concatenate)(w233, w232) -> (w231:string[])
        }
        n120 = Concatenate Strings(w210, w211, w189, "_Station_" ("시간 포맷 문자열 (%c)"), w188, "_Station : " ("시간 포맷 문자열 (%c)"), w187, w214, w213, "\r") -> (w204:string)
        n121 = Format Date/Time String(time format string (%c)="%Y_%m_%d_%H_" ("시간 포맷 문자열 (%c)")) -> (date/time string=w181:string)  [unwired: 2 in]
        n122 = Number To Decimal String(number=w199) -> (decimal integer string=w180:string)  [unwired: 1 in]
        n123 = Concatenate Strings(w181, w180) -> (→"Station_1_수신시작시간":string)
        n124 = Bundle By Name(cluster=w205, "로그기록"=w204, "RX_그래프_LED"=TRUE, "RX_그래프2_LED"=w202, "RX_그래프3_LED"=w202, "RX_그래프4_LED"=w202, "RX_그래프5_LED"=w202) -> (w201:T5)
        n125 = Build Array (concatenate)(w181, w180, w189, w188, w187, w184) -> (w183:string[])
        n126 = call "Save_teplete(Subvi).vi"("숫자형"=2, "배열"=w183) -> ()  [unwired: 10 in]
      }
      frame 2 {
        w409 = FALSE
        # "※ 2차원 벡터 -> 1차원 벡터"
        n127 = Subtract(x=w411, y=2000) -> (x-y=w458:i32)
        n128 = Format Date/Time String(time format string (%c)="%M" ("시간 포맷 문자열 (%c)")) -> (date/time string=w408:string)  [unwired: 2 in]
        n129 = call "Save_Log_File(Subvi).vi"("TX_Station"=w414, "RX_Station"=w435, "1D data"=w455) -> ()  [unwired: 7 in, 1 out]
        n130 = property on="Station_현황_TRX_Controller" class="MCListbox (엄격한)"() -> ("ItemNames"=w431:string[][])  [unwired: 2 in, 2 out]
        n131 = for {
          N: 4001 -> [_]
          tunnel: w458 -> [w635]
          shift-right: [w630] -> w456
          shift-left: dbl[] [] -> [w632]
          i -> [w629]
          n132 = Add(x=w635, y=w629) -> (x+y=w634:i32)
          n133 = Divide(x=w634, y=110000) -> (x/y=w631:dbl)
          n134 = Build Array (concatenate)(w632, w631) -> (w630:dbl[])
        }
        n135 = Decimal String To Number(string=w408) -> ()  [unwired: 2 in, 2 out]
        n136 = Unbundle By Name(w436) -> ("로그기록"=w442:string)
        n137 = Number To Decimal String(number=w414) -> (decimal integer string=w419:string)  [unwired: 1 in]
        n138 = Number To Decimal String(number=w435) -> (decimal integer string=w418:string)  [unwired: 1 in]
        n139 = Number To Decimal String(number=w411) -> (decimal integer string=w417:string)  [unwired: 1 in]
        n140 = Number To Decimal String(number=w438) -> (decimal integer string=w449:string)  [unwired: 1 in]
        n141 = Number To Decimal String(number=w437) -> (decimal integer string=w448:string)  [unwired: 1 in]
        n142 = case shown="5" w414 {
          tunnel: w413 -> [w464 w469 w505 w515 w554 w591]
          tunnel: [w463 w485 w506 w531 w570 w609] -> w410
          tunnel: [0 w471 0 w513 w552 w593] -> w412
          tunnel: w411 -> [_ w470 _ w514 w553 w592]
          tunnel: w406 -> [_ w465 _ w509 w548 w587]
          frame 0, Default {
            w462 = FALSE
            n143 = Bundle By Name(cluster=w464, "TX_그래프_LED"=w462, "TX_그래프2_LED"=w462, "TX_그래프3_LED"=w462, "TX_그래프4_LED"=w462, "TX_그래프5_LED"=w462) -> (w463:T6)
          }
          frame 1 {
            w486 = FALSE
            n144 = Unbundle By Name(w469) -> ("유속데이터흐름표_10분"=w472:string[][])
            n145 = Unbundle By Name(w469) -> ("유속데이터흐름표_30분"=w474:string[][])
            n146 = Unbundle By Name(w469) -> ("유속데이터흐름표_50분"=w473:string[][])
            n147 = Number To Decimal String(number=w470) -> (decimal integer string=w478:string)  [unwired: 1 in]
            n148 = Replace Array Subset(array=w472, new element=w478, index (row)=1 ("인덱스 (행)"), index (col)=0 ("비활성화된 인덱스 (열)")) -> (w477:string[][])
            n149 = Replace Array Subset(array=w474, new element=w478, index (row)=1 ("인덱스 (행)"), index (col)=0 ("비활성화된 인덱스 (열)")) -> (w476:string[][])
            n150 = Replace Array Subset(array=w473, new element=w478, index (row)=1 ("인덱스 (행)"), index (col)=0 ("비활성화된 인덱스 (열)")) -> (w475:string[][])
            n151 = case shown="0, 기본" w465 {
              tunnel: [0 10 30 50] -> w471
              tunnel: w477 -> [_ w494 _ _]
              tunnel: w476 -> [_ _ w497 _]
              tunnel: w475 -> [_ _ _ w500]
              tunnel: [w490 w494 w498 w502] -> w468
              tunnel: [w489 w493 w497 w501] -> w467
              tunnel: [w488 w492 w496 w500] -> w466
              tunnel: w474 -> [w489 w493 _ w501]
              tunnel: w473 -> [w488 w492 w496 _]
              tunnel: w472 -> [w490 _ w498 w502]
              frame 0, Default {
              }
              frame 10..15 {
              }
              frame 30..35 {
              }
              frame 50..55 {
              }
            }
            n152 = Bundle By Name(cluster=w469, "TX_그래프_LED"=TRUE, "TX_그래프2_LED"=w486, "TX_그래프3_LED"=w486, "TX_그래프4_LED"=w486, "TX_그래프5_LED"=w486, "유속데이터흐름표_10분"=w468, "유속데이터흐름표_30분"=w467, "유속데이터흐름표_50분"=w466) -> (w485:T6)
          }
          frame 2 {
            w507 = FALSE
            n153 = Bundle By Name(cluster=w505, "TX_그래프_LED"=w507, "TX_그래프2_LED"=TRUE, "TX_그래프3_LED"=w507, "TX_그래프4_LED"=w507, "TX_그래프5_LED"=w507) -> (w506:T6)
          }
          frame 3 {
            w529 = FALSE
            n154 = Unbundle By Name(w515) -> ("유속데이터흐름표_10분"=w528:string[][])
            n155 = Unbundle By Name(w515) -> ("유속데이터흐름표_30분"=w526:string[][])
            n156 = Unbundle By Name(w515) -> ("유속데이터흐름표_50분"=w527:string[][])
            n157 = Number To Decimal String(number=w514) -> (decimal integer string=w522:string)  [unwired: 1 in]
            n158 = Replace Array Subset(array=w528, new element=w522, index (row)=1 ("인덱스 (행)"), index (col)=2 ("비활성화된 인덱스 (열)")) -> (w523:string[][])
            n159 = Replace Array Subset(array=w526, new element=w522, index (row)=1 ("인덱스 (행)"), index (col)=2 ("비활성화된 인덱스 (열)")) -> (w524:string[][])
            n160 = Replace Array Subset(array=w527, new element=w522, index (row)=1 ("인덱스 (행)"), index (col)=2 ("비활성화된 인덱스 (열)")) -> (w525:string[][])
            n161 = case shown="50..55" w509 {
              tunnel: [0 12 32 52] -> w513
              tunnel: w523 -> [_ w538 _ _]
              tunnel: w524 -> [_ _ w541 _]
              tunnel: w525 -> [_ _ _ w544]
              tunnel: [w534 w538 w542 w546] -> w512
              tunnel: [w533 w537 w541 w545] -> w511
              tunnel: [w532 w536 w540 w544] -> w510
              tunnel: w526 -> [w533 w537 _ w545]
              tunnel: w527 -> [w532 w536 w540 _]
              tunnel: w528 -> [w534 _ w542 w546]
              frame 0, Default {
              }
              frame 10..15 {
              }
              frame 30..35 {
              }
              frame 50..55 {
              }
            }
            n162 = Bundle By Name(cluster=w515, "TX_그래프_LED"=w529, "TX_그래프2_LED"=w529, "TX_그래프3_LED"=TRUE, "TX_그래프4_LED"=w529, "TX_그래프5_LED"=w529, "유속데이터흐름표_10분"=w512, "유속데이터흐름표_30분"=w511, "유속데이터흐름표_50분"=w510) -> (w531:T6)
          }
          frame 4 {
            w568 = FALSE
            n163 = Unbundle By Name(w554) -> ("유속데이터흐름표_10분"=w567:string[][])
            n164 = Unbundle By Name(w554) -> ("유속데이터흐름표_30분"=w565:string[][])
            n165 = Unbundle By Name(w554) -> ("유속데이터흐름표_50분"=w566:string[][])
            n166 = Number To Decimal String(number=w553) -> (decimal integer string=w561:string)  [unwired: 1 in]
            n167 = Replace Array Subset(array=w567, new element=w561, index (row)=1 ("인덱스 (행)"), index (col)=3 ("비활성화된 인덱스 (열)")) -> (w562:string[][])
            n168 = Replace Array Subset(array=w565, new element=w561, index (row)=1 ("인덱스 (행)"), index (col)=3 ("비활성화된 인덱스 (열)")) -> (w563:string[][])
            n169 = Replace Array Subset(array=w566, new element=w561, index (row)=1 ("인덱스 (행)"), index (col)=3 ("비활성화된 인덱스 (열)")) -> (w564:string[][])
            n170 = case shown="10..15" w548 {
              tunnel: [0 13 33 53] -> w552
              tunnel: w562 -> [_ w577 _ _]
              tunnel: w563 -> [_ _ w580 _]
              tunnel: w564 -> [_ _ _ w583]
              tunnel: [w573 w577 w581 w585] -> w551
              tunnel: [w572 w576 w580 w584] -> w550
              tunnel: [w571 w575 w579 w583] -> w549
              tunnel: w565 -> [w572 w576 _ w584]
              tunnel: w566 -> [w571 w575 w579 _]
              tunnel: w567 -> [w573 _ w581 w585]
              frame 0, Default {
              }
              frame 10..15 {
              }
              frame 30..35 {
              }
              frame 50..55 {
              }
            }
            n171 = Bundle By Name(cluster=w554, "TX_그래프_LED"=w568, "TX_그래프2_LED"=w568, "TX_그래프3_LED"=w568, "TX_그래프4_LED"=TRUE, "TX_그래프5_LED"=w568, "유속데이터흐름표_10분"=w551, "유속데이터흐름표_30분"=w550, "유속데이터흐름표_50분"=w549) -> (w570:T6)
          }
          frame 5 {
            w607 = FALSE
            n172 = Unbundle By Name(w591) -> ("유속데이터흐름표_10분"=w606:string[][])
            n173 = Unbundle By Name(w591) -> ("유속데이터흐름표_30분"=w604:string[][])
            n174 = Unbundle By Name(w591) -> ("유속데이터흐름표_50분"=w605:string[][])
            n175 = Number To Decimal String(number=w592) -> (decimal integer string=w600:string)  [unwired: 1 in]
            n176 = Replace Array Subset(array=w606, new element=w600, index (row)=1 ("인덱스 (행)"), index (col)=4 ("비활성화된 인덱스 (열)")) -> (w601:string[][])
            n177 = Replace Array Subset(array=w604, new element=w600, index (row)=1 ("인덱스 (행)"), index (col)=4 ("비활성화된 인덱스 (열)")) -> (w602:string[][])
            n178 = Replace Array Subset(array=w605, new element=w600, index (row)=1 ("인덱스 (행)"), index (col)=4 ("비활성화된 인덱스 (열)")) -> (w603:string[][])
            n179 = case shown="0, 기본" w587 {
              tunnel: [0 14 34 54] -> w593
              tunnel: w601 -> [_ w616 _ _]
              tunnel: w602 -> [_ _ w619 _]
              tunnel: w603 -> [_ _ _ w622]
              tunnel: [w612 w616 w620 w624] -> w590
              tunnel: [w611 w615 w619 w623] -> w589
              tunnel: [w610 w614 w618 w622] -> w588
              tunnel: w604 -> [w611 w615 _ w623]
              tunnel: w605 -> [w610 w614 w618 _]
              tunnel: w606 -> [w612 _ w620 w624]
              frame 0, Default {
              }
              frame 10..15 {
              }
              frame 30..35 {
              }
              frame 50..55 {
              }
            }
            n180 = Bundle By Name(cluster=w591, "TX_그래프_LED"=w607, "TX_그래프2_LED"=w607, "TX_그래프3_LED"=w607, "TX_그래프4_LED"=w607, "TX_그래프5_LED"=TRUE, "유속데이터흐름표_10분"=w590, "유속데이터흐름표_30분"=w589, "유속데이터흐름표_50분"=w588) -> (w609:T6)
          }
        }
        n181 = Concatenate Strings("_Q_" ("시간 포맷 문자열 (%c)"), w449) -> (w446:string)
        n182 = Concatenate Strings("_Order : " ("시간 포맷 문자열 (%c)"), w448) -> (w445:string)
        n183 = Array Subset(array=w431, index (row)=0 ("인덱스"), length (row)=7 ("길이"), index (col)=0 ("인덱스"), length (col)=1 ("길이")) -> (w424:string[][])
        n184 = Format Date/Time String(time format string (%c)="%Y_%m_%d_%H_%M_" ("시간 포맷 문자열 (%c)")) -> (date/time string=w443:string)  [unwired: 2 in]
        n185 = Array Subset(array=w424, index (row)=3 ("인덱스"), length (row)=2 ("길이")) -> (w429:string[][])  [unwired: 2 in]
        n186 = Bundle(w456, w455) -> (→"Station_2":cluster{dbl[], i32[]})  [unwired: 1 in]
        n187 = for {
          tunnel: w429 -> [w627] mode=indexing
          shift-right: [w626] -> w416
          shift-left: string[] [] -> [w628]
          n188 = Build Array (concatenate)(w628, w627) -> (w626:string[])
        }
        n189 = Concatenate Strings(w442, w443, w419, "_Station_" ("시간 포맷 문자열 (%c)"), w418, "_Station : " ("시간 포맷 문자열 (%c)"), w417, w446, w445, "\r") -> (w441:string)
        n190 = Number To Decimal String(number=w412) -> (decimal integer string=w420:string)  [unwired: 1 in]
        n191 = Format Date/Time String(time format string (%c)="%Y_%m_%d_%H_" ("시간 포맷 문자열 (%c)")) -> (date/time string=w421:string)  [unwired: 2 in]
        n192 = Concatenate Strings(w421, w420) -> (→"Station_2_수신시작시간":string)
        n193 = Bundle By Name(cluster=w436, "로그기록"=w441, "RX_그래프_LED"=w409, "RX_그래프2_LED"=TRUE, "RX_그래프3_LED"=w409, "RX_그래프4_LED"=w409, "RX_그래프5_LED"=w409) -> (w439:T5)
        n194 = Build Array (concatenate)(w421, w420, w419, w418, w417, w416) -> (w415:string[])
        n195 = call "Save_teplete(Subvi).vi"("숫자형"=2, "배열"=w415) -> ()  [unwired: 10 in]
      }
      frame 3 {
        w665 = FALSE
        # "※2차원 벡터 -> 1차원 벡터"
        n196 = Format Date/Time String(time format string (%c)="%M" ("시간 포맷 문자열 (%c)")) -> (date/time string=w638:string)  [unwired: 2 in]
        n197 = Subtract(x=w641, y=2000) -> (x-y=w688:i32)
        n198 = call "Save_Log_File(Subvi).vi"("TX_Station"=w642, "RX_Station"=w669, "1D data"=w685) -> ()  [unwired: 7 in, 1 out]
        n199 = property on="Station_현황_TRX_Controller" class="MCListbox (엄격한)"() -> ("ItemNames"=w662:string[][])  [unwired: 2 in, 2 out]
        n200 = for {
          N: 4001 -> [_]
          tunnel: w688 -> [w865]
          shift-right: [w860] -> w686
          shift-left: dbl[] [] -> [w862]
          i -> [w859]
          n201 = Add(x=w865, y=w859) -> (x+y=w864:i32)
          n202 = Divide(x=w864, y=110000) -> (x/y=w861:dbl)
          n203 = Build Array (concatenate)(w862, w861) -> (w860:dbl[])
        }
        n204 = Decimal String To Number(string=w638) -> ()  [unwired: 2 in, 2 out]
        n205 = Unbundle By Name(w670) -> ("로그기록"=w673:string)
        n206 = Number To Decimal String(number=w642) -> (decimal integer string=w649:string)  [unwired: 1 in]
        n207 = Number To Decimal String(number=w669) -> (decimal integer string=w644:string)  [unwired: 1 in]
        n208 = Number To Decimal String(number=w641) -> (decimal integer string=w647:string)  [unwired: 1 in]
        n209 = Number To Decimal String(number=w668) -> (decimal integer string=w680:string)  [unwired: 1 in]
        n210 = Number To Decimal String(number=w667) -> (decimal integer string=w679:string)  [unwired: 1 in]
        n211 = case shown="5" w642 {
          tunnel: w643 -> [w694 w699 w739 w774 w784 w821]
          tunnel: [w693 w715 w754 w777 w800 w839] -> w639
          tunnel: [0 w701 w738 0 w782 w823] -> w640
          tunnel: w641 -> [_ w700 w740 _ w783 w822]
          tunnel: w636 -> [_ w695 w734 _ w778 w817]
          frame 0, Default {
            w692 = FALSE
            n212 = Bundle By Name(cluster=w694, "TX_그래프_LED"=w692, "TX_그래프2_LED"=w692, "TX_그래프3_LED"=w692, "TX_그래프4_LED"=w692, "TX_그래프5_LED"=w692) -> (w693:T6)
          }
          frame 1 {
            w716 = FALSE
            n213 = Unbundle By Name(w699) -> ("유속데이터흐름표_10분"=w702:string[][])
            n214 = Unbundle By Name(w699) -> ("유속데이터흐름표_30분"=w704:string[][])
            n215 = Unbundle By Name(w699) -> ("유속데이터흐름표_50분"=w703:string[][])
            n216 = Number To Decimal String(number=w700) -> (decimal integer string=w708:string)  [unwired: 1 in]
            n217 = Replace Array Subset(array=w702, new element=w708, index (row)=2 ("인덱스 (행)"), index (col)=0 ("비활성화된 인덱스 (열)")) -> (w707:string[][])
            n218 = Replace Array Subset(array=w704, new element=w708, index (row)=2 ("인덱스 (행)"), index (col)=0 ("비활성화된 인덱스 (열)")) -> (w706:string[][])
            n219 = Replace Array Subset(array=w703, new element=w708, index (row)=2 ("인덱스 (행)"), index (col)=0 ("비활성화된 인덱스 (열)")) -> (w705:string[][])
            n220 = case shown="10..15" w695 {
              tunnel: [0 10 30 50] -> w701
              tunnel: w707 -> [_ w724 _ _]
              tunnel: w706 -> [_ _ w727 _]
              tunnel: w705 -> [_ _ _ w730]
              tunnel: [w720 w724 w728 w732] -> w698
              tunnel: [w719 w723 w727 w731] -> w697
              tunnel: [w718 w722 w726 w730] -> w696
              tunnel: w704 -> [w719 w723 _ w731]
              tunnel: w703 -> [w718 w722 w726 _]
              tunnel: w702 -> [w720 _ w728 w732]
              frame 0, Default {
              }
              frame 10..15 {
              }
              frame 30..35 {
              }
              frame 50..55 {
              }
            }
            n221 = Bundle By Name(cluster=w699, "TX_그래프_LED"=TRUE, "TX_그래프2_LED"=w716, "TX_그래프3_LED"=w716, "TX_그래프4_LED"=w716, "TX_그래프5_LED"=w716, "유속데이터흐름표_10분"=w698, "유속데이터흐름표_30분"=w697, "유속데이터흐름표_50분"=w696) -> (w715:T6)
          }
          frame 2 {
            w755 = FALSE
            n222 = Unbundle By Name(w739) -> ("유속데이터흐름표_10분"=w741:string[][])
            n223 = Unbundle By Name(w739) -> ("유속데이터흐름표_30분"=w743:string[][])
            n224 = Unbundle By Name(w739) -> ("유속데이터흐름표_50분"=w742:string[][])
            n225 = Number To Decimal String(number=w740) -> (decimal integer string=w747:string)  [unwired: 1 in]
            n226 = Replace Array Subset(array=w741, new element=w747, index (row)=2 ("인덱스 (행)"), index (col)=1 ("비활성화된 인덱스 (열)")) -> (w746:string[][])
            n227 = Replace Array Subset(array=w743, new element=w747, index (row)=2 ("인덱스 (행)"), index (col)=1 ("비활성화된 인덱스 (열)")) -> (w745:string[][])
            n228 = Replace Array Subset(array=w742, new element=w747, index (row)=2 ("인덱스 (행)"), index (col)=1 ("비활성화된 인덱스 (열)")) -> (w744:string[][])
            n229 = case shown="50..55" w734 {
              tunnel: [0 11 31 51] -> w738
              tunnel: w746 -> [_ w763 _ _]
              tunnel: w745 -> [_ _ w766 _]
              tunnel: w744 -> [_ _ _ w769]
              tunnel: [w759 w763 w767 w771] -> w737
              tunnel: [w758 w762 w766 w770] -> w736
              tunnel: [w757 w761 w765 w769] -> w735
              tunnel: w743 -> [w758 w762 _ w770]
              tunnel: w742 -> [w757 w761 w765 _]
              tunnel: w741 -> [w759 _ w767 w771]
              frame 0, Default {
              }
              frame 10..15 {
              }
              frame 30..35 {
              }
              frame 50..55 {
              }
            }
            n230 = Bundle By Name(cluster=w739, "TX_그래프_LED"=w755, "TX_그래프2_LED"=TRUE, "TX_그래프3_LED"=w755, "TX_그래프4_LED"=w755, "TX_그래프5_LED"=w755, "유속데이터흐름표_10분"=w737, "유속데이터흐름표_30분"=w736, "유속데이터흐름표_50분"=w735) -> (w754:T6)
          }
          frame 3 {
            w775 = FALSE
            n231 = Bundle By Name(cluster=w774, "TX_그래프_LED"=w775, "TX_그래프2_LED"=w775, "TX_그래프3_LED"=TRUE, "TX_그래프4_LED"=w775, "TX_그래프5_LED"=w775) -> (w777:T6)
          }
          frame 4 {
            w798 = FALSE
            n232 = Unbundle By Name(w784) -> ("유속데이터흐름표_10분"=w797:string[][])
            n233 = Unbundle By Name(w784) -> ("유속데이터흐름표_30분"=w795:string[][])
            n234 = Unbundle By Name(w784) -> ("유속데이터흐름표_50분"=w796:string[][])
            n235 = Number To Decimal String(number=w783) -> (decimal integer string=w791:string)  [unwired: 1 in]
            n236 = Replace Array Subset(array=w797, new element=w791, index (row)=2 ("인덱스 (행)"), index (col)=3 ("비활성화된 인덱스 (열)")) -> (w792:string[][])
            n237 = Replace Array Subset(array=w795, new element=w791, index (row)=2 ("인덱스 (행)"), index (col)=3 ("비활성화된 인덱스 (열)")) -> (w793:string[][])
            n238 = Replace Array Subset(array=w796, new element=w791, index (row)=2 ("인덱스 (행)"), index (col)=3 ("비활성화된 인덱스 (열)")) -> (w794:string[][])
            n239 = case shown="10..15" w778 {
              tunnel: [0 13 33 53] -> w782
              tunnel: w792 -> [_ w807 _ _]
              tunnel: w793 -> [_ _ w810 _]
              tunnel: w794 -> [_ _ _ w813]
              tunnel: [w803 w807 w811 w815] -> w781
              tunnel: [w802 w806 w810 w814] -> w780
              tunnel: [w801 w805 w809 w813] -> w779
              tunnel: w795 -> [w802 w806 _ w814]
              tunnel: w796 -> [w801 w805 w809 _]
              tunnel: w797 -> [w803 _ w811 w815]
              frame 0, Default {
              }
              frame 10..15 {
              }
              frame 30..35 {
              }
              frame 50..55 {
              }
            }
            n240 = Bundle By Name(cluster=w784, "TX_그래프_LED"=w798, "TX_그래프2_LED"=w798, "TX_그래프3_LED"=w798, "TX_그래프4_LED"=TRUE, "TX_그래프5_LED"=w798, "유속데이터흐름표_10분"=w781, "유속데이터흐름표_30분"=w780, "유속데이터흐름표_50분"=w779) -> (w800:T6)
          }
          frame 5 {
            w837 = FALSE
            n241 = Unbundle By Name(w821) -> ("유속데이터흐름표_10분"=w836:string[][])
            n242 = Unbundle By Name(w821) -> ("유속데이터흐름표_30분"=w834:string[][])
            n243 = Unbundle By Name(w821) -> ("유속데이터흐름표_50분"=w835:string[][])
            n244 = Number To Decimal String(number=w822) -> (decimal integer string=w830:string)  [unwired: 1 in]
            n245 = Replace Array Subset(array=w836, new element=w830, index (row)=2 ("인덱스 (행)"), index (col)=4 ("비활성화된 인덱스 (열)")) -> (w831:string[][])
            n246 = Replace Array Subset(array=w834, new element=w830, index (row)=2 ("인덱스 (행)"), index (col)=4 ("비활성화된 인덱스 (열)")) -> (w832:string[][])
            n247 = Replace Array Subset(array=w835, new element=w830, index (row)=2 ("인덱스 (행)"), index (col)=4 ("비활성화된 인덱스 (열)")) -> (w833:string[][])
            n248 = case shown="10..15" w817 {
              tunnel: [0 14 34 54] -> w823
              tunnel: w831 -> [_ w846 _ _]
              tunnel: w832 -> [_ _ w849 _]
              tunnel: w833 -> [_ _ _ w852]
              tunnel: [w842 w846 w850 w854] -> w820
              tunnel: [w841 w845 w849 w853] -> w819
              tunnel: [w840 w844 w848 w852] -> w818
              tunnel: w834 -> [w841 w845 _ w853]
              tunnel: w835 -> [w840 w844 w848 _]
              tunnel: w836 -> [w842 _ w850 w854]
              frame 0, Default {
              }
              frame 10..15 {
              }
              frame 30..35 {
              }
              frame 50..55 {
              }
            }
            n249 = Bundle By Name(cluster=w821, "TX_그래프_LED"=w837, "TX_그래프2_LED"=w837, "TX_그래프3_LED"=w837, "TX_그래프4_LED"=w837, "TX_그래프5_LED"=TRUE, "유속데이터흐름표_10분"=w820, "유속데이터흐름표_30분"=w819, "유속데이터흐름표_50분"=w818) -> (w839:T6)
          }
        }
        n250 = Concatenate Strings("_Q_" ("시간 포맷 문자열 (%c)"), w680) -> (w677:string)
        n251 = Concatenate Strings("_Order : " ("시간 포맷 문자열 (%c)"), w679) -> (w676:string)
        n252 = Array Subset(array=w662, index (row)=0 ("인덱스"), length (row)=7 ("길이"), index (col)=0 ("인덱스"), length (col)=1 ("길이")) -> (w655:string[][])
        n253 = Format Date/Time String(time format string (%c)="%Y_%m_%d_%H_%M_" ("시간 포맷 문자열 (%c)")) -> (date/time string=w674:string)  [unwired: 2 in]
        n254 = Array Subset(array=w655, index (row)=3 ("인덱스"), length (row)=2 ("길이")) -> (w660:string[][])  [unwired: 2 in]
        n255 = Bundle(w686, w685) -> (→"Station_3":cluster{dbl[], i32[]})  [unwired: 1 in]
        n256 = for {
          tunnel: w660 -> [w857] mode=indexing
          shift-right: [w856] -> w646
          shift-left: string[] [] -> [w858]
          n257 = Build Array (concatenate)(w858, w857) -> (w856:string[])
        }
        n258 = Concatenate Strings(w673, w674, w649, "_Station_" ("시간 포맷 문자열 (%c)"), w644, "_Station : " ("시간 포맷 문자열 (%c)"), w647, w677, w676, "\r") -> (w672:string)
        n259 = Number To Decimal String(number=w640) -> (decimal integer string=w650:string)  [unwired: 1 in]
        n260 = Format Date/Time String(time format string (%c)="%Y_%m_%d_%H_" ("시간 포맷 문자열 (%c)")) -> (date/time string=w651:string)  [unwired: 2 in]
        n261 = Concatenate Strings(w651, w650) -> (→"Station_3_수신시작시간":string)
        n262 = Bundle By Name(cluster=w670, "로그기록"=w672, "RX_그래프_LED"=w665, "RX_그래프2_LED"=w665, "RX_그래프3_LED"=TRUE, "RX_그래프4_LED"=w665, "RX_그래프5_LED"=w665) -> (w671:T5)
        n263 = Build Array (concatenate)(w651, w650, w649, w644, w647, w646) -> (w645:string[])
        n264 = call "Save_teplete(Subvi).vi"("숫자형"=2, "배열"=w645) -> ()  [unwired: 10 in]
      }
      frame 4 {
        w894 = FALSE
        # "※2차원 벡터 -> 1차원 벡터"
        n265 = Format Date/Time String(time format string (%c)="%M" ("시간 포맷 문자열 (%c)")) -> (date/time string=w868:string)  [unwired: 2 in]
        n266 = Subtract(x=w869, y=2000) -> (x-y=w918:i32)
        n267 = Decimal String To Number(string=w868) -> ()  [unwired: 2 in, 2 out]
        n268 = call "Save_Log_File(Subvi).vi"("TX_Station"=w870, "RX_Station"=w898, "1D data"=w915) -> ()  [unwired: 7 in, 1 out]
        n269 = Unbundle By Name(w899) -> ("로그기록"=w902:string)
        n270 = Number To Decimal String(number=w870) -> (decimal integer string=w877:string)  [unwired: 1 in]
        n271 = Number To Decimal String(number=w898) -> (decimal integer string=w876:string)  [unwired: 1 in]
        n272 = Number To Decimal String(number=w869) -> (decimal integer string=w875:string)  [unwired: 1 in]
        n273 = Number To Decimal String(number=w897) -> (decimal integer string=w909:string)  [unwired: 1 in]
        n274 = Number To Decimal String(number=w896) -> (decimal integer string=w908:string)  [unwired: 1 in]
        n275 = for {
          N: 4001 -> [_]
          tunnel: w918 -> [w1095]
          shift-right: [w1090] -> w916
          shift-left: dbl[] [] -> [w1092]
          i -> [w1089]
          n276 = Add(x=w1095, y=w1089) -> (x+y=w1094:i32)
          n277 = Divide(x=w1094, y=110000) -> (x/y=w1091:dbl)
          n278 = Build Array (concatenate)(w1092, w1091) -> (w1090:dbl[])
        }
        n279 = case shown="1" w870 {
          tunnel: [w924 w945 w984 w1025 w1046 w1069] -> w872
          tunnel: [0 w934 w973 w1010 0 w1056] -> w873
          tunnel: w871 -> [w921 w930 w969 w1012 w1043 w1052]
          tunnel: w869 -> [_ w929 w968 w1011 _ w1051]
          tunnel: w866 -> [_ w925 w964 w1003 _ w1047]
          frame 0, Default {
            w923 = FALSE
            n280 = Bundle By Name(cluster=w921, "TX_그래프_LED"=w923, "TX_그래프2_LED"=w923, "TX_그래프3_LED"=w923, "TX_그래프4_LED"=w923, "TX_그래프5_LED"=w923) -> (w924:T6)
          }
          frame 1 {
            w946 = FALSE
            n281 = Unbundle By Name(w930) -> ("유속데이터흐름표_10분"=w928:string[][])
            n282 = Unbundle By Name(w930) -> ("유속데이터흐름표_30분"=w927:string[][])
            n283 = Unbundle By Name(w930) -> ("유속데이터흐름표_50분"=w926:string[][])
            n284 = Number To Decimal String(number=w929) -> (decimal integer string=w938:string)  [unwired: 1 in]
            n285 = Replace Array Subset(array=w928, new element=w938, index (row)=3 ("인덱스 (행)"), index (col)=0 ("비활성화된 인덱스 (열)")) -> (w937:string[][])
            n286 = Replace Array Subset(array=w927, new element=w938, index (row)=3 ("인덱스 (행)"), index (col)=0 ("비활성화된 인덱스 (열)")) -> (w936:string[][])
            n287 = Replace Array Subset(array=w926, new element=w938, index (row)=3 ("인덱스 (행)"), index (col)=0 ("비활성화된 인덱스 (열)")) -> (w935:string[][])
            n288 = case shown="50..55" w925 {
              tunnel: [0 10 30 50] -> w934
              tunnel: w937 -> [_ w954 _ _]
              tunnel: w936 -> [_ _ w958 _]
              tunnel: w935 -> [_ _ _ w962]
              tunnel: [w950 w954 w957 w961] -> w933
              tunnel: [w949 w953 w958 w960] -> w932
              tunnel: [w948 w952 w956 w962] -> w931
              tunnel: w927 -> [w949 w953 _ w960]
              tunnel: w926 -> [w948 w952 w956 _]
              tunnel: w928 -> [w950 _ w957 w961]
              frame 0, Default {
              }
              frame 10..15 {
              }
              frame 30..35 {
              }
              frame 50..55 {
              }
            }
            n289 = Bundle By Name(cluster=w930, "TX_그래프_LED"=TRUE, "TX_그래프2_LED"=w946, "TX_그래프3_LED"=w946, "TX_그래프4_LED"=w946, "TX_그래프5_LED"=w946, "유속데이터흐름표_10분"=w933, "유속데이터흐름표_30분"=w932, "유속데이터흐름표_50분"=w931) -> (w945:T6)
          }
          frame 2 {
            w985 = FALSE
            n290 = Unbundle By Name(w969) -> ("유속데이터흐름표_10분"=w967:string[][])
            n291 = Unbundle By Name(w969) -> ("유속데이터흐름표_30분"=w966:string[][])
            n292 = Unbundle By Name(w969) -> ("유속데이터흐름표_50분"=w965:string[][])
            n293 = Number To Decimal String(number=w968) -> (decimal integer string=w977:string)  [unwired: 1 in]
            n294 = Replace Array Subset(array=w967, new element=w977, index (row)=3 ("인덱스 (행)"), index (col)=1 ("비활성화된 인덱스 (열)")) -> (w976:string[][])
            n295 = Replace Array Subset(array=w966, new element=w977, index (row)=3 ("인덱스 (행)"), index (col)=1 ("비활성화된 인덱스 (열)")) -> (w975:string[][])
            n296 = Replace Array Subset(array=w965, new element=w977, index (row)=3 ("인덱스 (행)"), index (col)=1 ("비활성화된 인덱스 (열)")) -> (w974:string[][])
            n297 = case shown="10..15" w964 {
              tunnel: [0 11 31 51] -> w973
              tunnel: w976 -> [_ w993 _ _]
              tunnel: w975 -> [_ _ w997 _]
              tunnel: w974 -> [_ _ _ w1001]
              tunnel: [w989 w993 w996 w1000] -> w972
              tunnel: [w988 w992 w997 w999] -> w971
              tunnel: [w987 w991 w995 w1001] -> w970
              tunnel: w966 -> [w988 w992 _ w999]
              tunnel: w965 -> [w987 w991 w995 _]
              tunnel: w967 -> [w989 _ w996 w1000]
              frame 0, Default {
              }
              frame 10..15 {
              }
              frame 30..35 {
              }
              frame 50..55 {
              }
            }
            n298 = Bundle By Name(cluster=w969, "TX_그래프_LED"=w985, "TX_그래프2_LED"=TRUE, "TX_그래프3_LED"=w985, "TX_그래프4_LED"=w985, "TX_그래프5_LED"=w985, "유속데이터흐름표_10분"=w972, "유속데이터흐름표_30분"=w971, "유속데이터흐름표_50분"=w970) -> (w984:T6)
          }
          frame 3 {
            w1023 = FALSE
            n299 = Unbundle By Name(w1012) -> ("유속데이터흐름표_10분"=w1006:string[][])
            n300 = Unbundle By Name(w1012) -> ("유속데이터흐름표_30분"=w1005:string[][])
            n301 = Unbundle By Name(w1012) -> ("유속데이터흐름표_50분"=w1004:string[][])
            n302 = Number To Decimal String(number=w1011) -> (decimal integer string=w1016:string)  [unwired: 1 in]
            n303 = Replace Array Subset(array=w1006, new element=w1016, index (row)=3 ("인덱스 (행)"), index (col)=2 ("비활성화된 인덱스 (열)")) -> (w1015:string[][])
            n304 = Replace Array Subset(array=w1005, new element=w1016, index (row)=3 ("인덱스 (행)"), index (col)=2 ("비활성화된 인덱스 (열)")) -> (w1014:string[][])
            n305 = Replace Array Subset(array=w1004, new element=w1016, index (row)=3 ("인덱스 (행)"), index (col)=2 ("비활성화된 인덱스 (열)")) -> (w1013:string[][])
            n306 = case shown="10..15" w1003 {
              tunnel: [0 12 32 52] -> w1010
              tunnel: w1015 -> [_ w1032 _ _]
              tunnel: w1014 -> [_ _ w1036 _]
              tunnel: w1013 -> [_ _ _ w1040]
              tunnel: [w1028 w1032 w1035 w1039] -> w1009
              tunnel: [w1027 w1031 w1036 w1038] -> w1008
              tunnel: [w1026 w1030 w1034 w1040] -> w1007
              tunnel: w1005 -> [w1027 w1031 _ w1038]
              tunnel: w1004 -> [w1026 w1030 w1034 _]
              tunnel: w1006 -> [w1028 _ w1035 w1039]
              frame 0, Default {
              }
              frame 10..15 {
              }
              frame 30..35 {
              }
              frame 50..55 {
              }
            }
            n307 = Bundle By Name(cluster=w1012, "TX_그래프_LED"=w1023, "TX_그래프2_LED"=w1023, "TX_그래프3_LED"=TRUE, "TX_그래프4_LED"=w1023, "TX_그래프5_LED"=w1023, "유속데이터흐름표_10분"=w1009, "유속데이터흐름표_30분"=w1008, "유속데이터흐름표_50분"=w1007) -> (w1025:T6)
          }
          frame 4 {
            w1044 = FALSE
            n308 = Bundle By Name(cluster=w1043, "TX_그래프_LED"=w1044, "TX_그래프2_LED"=w1044, "TX_그래프3_LED"=w1044, "TX_그래프4_LED"=TRUE, "TX_그래프5_LED"=w1044) -> (w1046:T6)
          }
          frame 5 {
            w1067 = FALSE
            n309 = Unbundle By Name(w1052) -> ("유속데이터흐름표_10분"=w1050:string[][])
            n310 = Unbundle By Name(w1052) -> ("유속데이터흐름표_30분"=w1049:string[][])
            n311 = Unbundle By Name(w1052) -> ("유속데이터흐름표_50분"=w1048:string[][])
            n312 = Number To Decimal String(number=w1051) -> (decimal integer string=w1063:string)  [unwired: 1 in]
            n313 = Replace Array Subset(array=w1050, new element=w1063, index (row)=3 ("인덱스 (행)"), index (col)=4 ("비활성화된 인덱스 (열)")) -> (w1064:string[][])
            n314 = Replace Array Subset(array=w1049, new element=w1063, index (row)=3 ("인덱스 (행)"), index (col)=4 ("비활성화된 인덱스 (열)")) -> (w1065:string[][])
            n315 = Replace Array Subset(array=w1048, new element=w1063, index (row)=3 ("인덱스 (행)"), index (col)=4 ("비활성화된 인덱스 (열)")) -> (w1066:string[][])
            n316 = case shown="10..15" w1047 {
              tunnel: [0 14 34 54] -> w1056
              tunnel: w1064 -> [_ w1076 _ _]
              tunnel: w1065 -> [_ _ w1080 _]
              tunnel: w1066 -> [_ _ _ w1084]
              tunnel: [w1072 w1076 w1079 w1083] -> w1055
              tunnel: [w1071 w1075 w1080 w1082] -> w1054
              tunnel: [w1070 w1074 w1078 w1084] -> w1053
              tunnel: w1049 -> [w1071 w1075 _ w1082]
              tunnel: w1048 -> [w1070 w1074 w1078 _]
              tunnel: w1050 -> [w1072 _ w1079 w1083]
              frame 0, Default {
              }
              frame 10..15 {
              }
              frame 30..35 {
              }
              frame 50..55 {
              }
            }
            n317 = Bundle By Name(cluster=w1052, "TX_그래프_LED"=w1067, "TX_그래프2_LED"=w1067, "TX_그래프3_LED"=w1067, "TX_그래프4_LED"=w1067, "TX_그래프5_LED"=TRUE, "유속데이터흐름표_10분"=w1055, "유속데이터흐름표_30분"=w1054, "유속데이터흐름표_50분"=w1053) -> (w1069:T6)
          }
        }
        n318 = Concatenate Strings("_Q_" ("시간 포맷 문자열 (%c)"), w909) -> (w906:string)
        n319 = Concatenate Strings("_Order : " ("시간 포맷 문자열 (%c)"), w908) -> (w905:string)
        n320 = Format Date/Time String(time format string (%c)="%Y_%m_%d_%H_%M_" ("시간 포맷 문자열 (%c)")) -> (date/time string=w903:string)  [unwired: 2 in]
        n321 = Bundle(w916, w915) -> (→"Station_4":cluster{dbl[], i32[]})  [unwired: 1 in]
        n322 = Concatenate Strings(w902, w903, w877, "_Station_" ("시간 포맷 문자열 (%c)"), w876, "_Station : " ("시간 포맷 문자열 (%c)"), w875, w906, w905, "\r") -> (w901:string)
        n323 = property on="Station_현황_TRX_Controller" class="MCListbox (엄격한)"() -> ("ItemNames"=w891:string[][])  [unwired: 2 in, 2 out]
        n324 = Array Subset(array=w891, index (row)=0 ("인덱스"), length (row)=7 ("길이"), index (col)=0 ("인덱스"), length (col)=1 ("길이")) -> (w884:string[][])
        n325 = Array Subset(array=w884, index (row)=3 ("인덱스"), length (row)=2 ("길이")) -> (w889:string[][])  [unwired: 2 in]
        n326 = for {
          tunnel: w889 -> [w1087] mode=indexing
          shift-right: [w1086] -> w874
          shift-left: string[] [] -> [w1088]
          n327 = Build Array (concatenate)(w1088, w1087) -> (w1086:string[])
        }
        n328 = Format Date/Time String(time format string (%c)="%Y_%m_%d_%H_" ("시간 포맷 문자열 (%c)")) -> (date/time string=w880:string)  [unwired: 2 in]
        n329 = Number To Decimal String(number=w873) -> (decimal integer string=w879:string)  [unwired: 1 in]
        n330 = Concatenate Strings(w880, w879) -> (→"Station_4_수신시작시간":string)
        n331 = Bundle By Name(cluster=w899, "로그기록"=w901, "RX_그래프_LED"=w894, "RX_그래프2_LED"=w894, "RX_그래프3_LED"=w894, "RX_그래프4_LED"=TRUE, "RX_그래프5_LED"=w894) -> (w900:T5)
        n332 = Build Array (concatenate)(w880, w879, w877, w876, w875, w874) -> (w878:string[])
        n333 = call "Save_teplete(Subvi).vi"("숫자형"=2, "배열"=w878) -> ()  [unwired: 10 in]
      }
      frame 5 {
        w1124 = FALSE
        # "※2차원 벡터 -> 1차원 벡터"
        n334 = Format Date/Time String(time format string (%c)="%M" ("시간 포맷 문자열 (%c)")) -> (date/time string=w1098:string)  [unwired: 2 in]
        n335 = property on="Station_현황_TRX_Controller" class="MCListbox (엄격한)"() -> ("ItemNames"=w1121:string[][])  [unwired: 2 in, 2 out]
        n336 = Subtract(x=w1099, y=2000) -> (x-y=w1148:i32)
        n337 = Decimal String To Number(string=w1098) -> ()  [unwired: 2 in, 2 out]
        n338 = call "Save_Log_File(Subvi).vi"("TX_Station"=w1100, "RX_Station"=w1128, "1D data"=w1145) -> ()  [unwired: 7 in, 1 out]
        n339 = for {
          N: 4001 -> [_]
          tunnel: w1148 -> [w1325]
          shift-right: [w1320] -> w1146
          shift-left: dbl[] [] -> [w1322]
          i -> [w1319]
          n340 = Add(x=w1325, y=w1319) -> (x+y=w1324:i32)
          n341 = Divide(x=w1324, y=110000) -> (x/y=w1321:dbl)
          n342 = Build Array (concatenate)(w1322, w1321) -> (w1320:dbl[])
        }
        n343 = Unbundle By Name(w1129) -> ("로그기록"=w1132:string)
        n344 = Number To Decimal String(number=w1100) -> (decimal integer string=w1108:string)  [unwired: 1 in]
        n345 = case shown="5" w1100 {
          tunnel: [w1154 w1175 w1214 w1255 w1294 w1315] -> w1102
          tunnel: [0 w1164 w1203 w1240 w1279 0] -> w1103
          tunnel: w1101 -> [w1151 w1160 w1199 w1242 w1281 w1312]
          tunnel: w1099 -> [_ w1159 w1198 w1241 w1280 _]
          tunnel: w1096 -> [_ w1155 w1194 w1233 w1272 _]
          frame 0, Default {
            w1153 = FALSE
            n346 = Bundle By Name(cluster=w1151, "TX_그래프_LED"=w1153, "TX_그래프2_LED"=w1153, "TX_그래프3_LED"=w1153, "TX_그래프4_LED"=w1153, "TX_그래프5_LED"=w1153) -> (w1154:T6)
          }
          frame 1 {
            w1176 = FALSE
            n347 = Unbundle By Name(w1160) -> ("유속데이터흐름표_10분"=w1158:string[][])
            n348 = Unbundle By Name(w1160) -> ("유속데이터흐름표_30분"=w1157:string[][])
            n349 = Unbundle By Name(w1160) -> ("유속데이터흐름표_50분"=w1156:string[][])
            n350 = Number To Decimal String(number=w1159) -> (decimal integer string=w1168:string)  [unwired: 1 in]
            n351 = Replace Array Subset(array=w1158, new element=w1168, index (row)=4 ("인덱스 (행)"), index (col)=0 ("비활성화된 인덱스 (열)")) -> (w1167:string[][])
            n352 = Replace Array Subset(array=w1157, new element=w1168, index (row)=4 ("인덱스 (행)"), index (col)=0 ("비활성화된 인덱스 (열)")) -> (w1166:string[][])
            n353 = Replace Array Subset(array=w1156, new element=w1168, index (row)=4 ("인덱스 (행)"), index (col)=0 ("비활성화된 인덱스 (열)")) -> (w1165:string[][])
            n354 = case shown="50..55" w1155 {
              tunnel: [0 10 30 50] -> w1164
              tunnel: w1167 -> [_ w1184 _ _]
              tunnel: w1166 -> [_ _ w1188 _]
              tunnel: w1165 -> [_ _ _ w1192]
              tunnel: [w1180 w1184 w1187 w1191] -> w1163
              tunnel: [w1179 w1183 w1188 w1190] -> w1162
              tunnel: [w1178 w1182 w1186 w1192] -> w1161
              tunnel: w1157 -> [w1179 w1183 _ w1190]
              tunnel: w1156 -> [w1178 w1182 w1186 _]
              tunnel: w1158 -> [w1180 _ w1187 w1191]
              frame 0, Default {
              }
              frame 10..15 {
              }
              frame 30..35 {
              }
              frame 50..55 {
              }
            }
            n355 = Bundle By Name(cluster=w1160, "TX_그래프_LED"=TRUE, "TX_그래프2_LED"=w1176, "TX_그래프3_LED"=w1176, "TX_그래프4_LED"=w1176, "TX_그래프5_LED"=w1176, "유속데이터흐름표_10분"=w1163, "유속데이터흐름표_30분"=w1162, "유속데이터흐름표_50분"=w1161) -> (w1175:T6)
          }
          frame 2 {
            w1215 = FALSE
            n356 = Unbundle By Name(w1199) -> ("유속데이터흐름표_10분"=w1197:string[][])
            n357 = Unbundle By Name(w1199) -> ("유속데이터흐름표_30분"=w1196:string[][])
            n358 = Unbundle By Name(w1199) -> ("유속데이터흐름표_50분"=w1195:string[][])
            n359 = Number To Decimal String(number=w1198) -> (decimal integer string=w1207:string)  [unwired: 1 in]
            n360 = Replace Array Subset(array=w1197, new element=w1207, index (row)=4 ("인덱스 (행)"), index (col)=1 ("비활성화된 인덱스 (열)")) -> (w1206:string[][])
            n361 = Replace Array Subset(array=w1196, new element=w1207, index (row)=4 ("인덱스 (행)"), index (col)=1 ("비활성화된 인덱스 (열)")) -> (w1205:string[][])
            n362 = Replace Array Subset(array=w1195, new element=w1207, index (row)=4 ("인덱스 (행)"), index (col)=1 ("비활성화된 인덱스 (열)")) -> (w1204:string[][])
            n363 = case shown="50..55" w1194 {
              tunnel: [0 11 31 51] -> w1203
              tunnel: w1206 -> [_ w1223 _ _]
              tunnel: w1205 -> [_ _ w1227 _]
              tunnel: w1204 -> [_ _ _ w1231]
              tunnel: [w1219 w1223 w1226 w1230] -> w1202
              tunnel: [w1218 w1222 w1227 w1229] -> w1201
              tunnel: [w1217 w1221 w1225 w1231] -> w1200
              tunnel: w1196 -> [w1218 w1222 _ w1229]
              tunnel: w1195 -> [w1217 w1221 w1225 _]
              tunnel: w1197 -> [w1219 _ w1226 w1230]
              frame 0, Default {
              }
              frame 10..15 {
              }
              frame 30..35 {
              }
              frame 50..55 {
              }
            }
            n364 = Bundle By Name(cluster=w1199, "TX_그래프_LED"=w1215, "TX_그래프2_LED"=TRUE, "TX_그래프3_LED"=w1215, "TX_그래프4_LED"=w1215, "TX_그래프5_LED"=w1215, "유속데이터흐름표_10분"=w1202, "유속데이터흐름표_30분"=w1201, "유속데이터흐름표_50분"=w1200) -> (w1214:T6)
          }
          frame 3 {
            w1253 = FALSE
            n365 = Unbundle By Name(w1242) -> ("유속데이터흐름표_10분"=w1236:string[][])
            n366 = Unbundle By Name(w1242) -> ("유속데이터흐름표_30분"=w1235:string[][])
            n367 = Unbundle By Name(w1242) -> ("유속데이터흐름표_50분"=w1234:string[][])
            n368 = Number To Decimal String(number=w1241) -> (decimal integer string=w1246:string)  [unwired: 1 in]
            n369 = Replace Array Subset(array=w1236, new element=w1246, index (row)=4 ("인덱스 (행)"), index (col)=2 ("비활성화된 인덱스 (열)")) -> (w1245:string[][])
            n370 = Replace Array Subset(array=w1235, new element=w1246, index (row)=4 ("인덱스 (행)"), index (col)=2 ("비활성화된 인덱스 (열)")) -> (w1244:string[][])
            n371 = Replace Array Subset(array=w1234, new element=w1246, index (row)=4 ("인덱스 (행)"), index (col)=2 ("비활성화된 인덱스 (열)")) -> (w1243:string[][])
            n372 = case shown="10..15" w1233 {
              tunnel: [0 12 32 52] -> w1240
              tunnel: w1245 -> [_ w1262 _ _]
              tunnel: w1244 -> [_ _ w1266 _]
              tunnel: w1243 -> [_ _ _ w1270]
              tunnel: [w1258 w1262 w1265 w1269] -> w1239
              tunnel: [w1257 w1261 w1266 w1268] -> w1238
              tunnel: [w1256 w1260 w1264 w1270] -> w1237
              tunnel: w1235 -> [w1257 w1261 _ w1268]
              tunnel: w1234 -> [w1256 w1260 w1264 _]
              tunnel: w1236 -> [w1258 _ w1265 w1269]
              frame 0, Default {
              }
              frame 10..15 {
              }
              frame 30..35 {
              }
              frame 50..55 {
              }
            }
            n373 = Bundle By Name(cluster=w1242, "TX_그래프_LED"=w1253, "TX_그래프2_LED"=w1253, "TX_그래프3_LED"=TRUE, "TX_그래프4_LED"=w1253, "TX_그래프5_LED"=w1253, "유속데이터흐름표_10분"=w1239, "유속데이터흐름표_30분"=w1238, "유속데이터흐름표_50분"=w1237) -> (w1255:T6)
          }
          frame 4 {
            w1292 = FALSE
            n374 = Unbundle By Name(w1281) -> ("유속데이터흐름표_10분"=w1275:string[][])
            n375 = Unbundle By Name(w1281) -> ("유속데이터흐름표_30분"=w1274:string[][])
            n376 = Unbundle By Name(w1281) -> ("유속데이터흐름표_50분"=w1273:string[][])
            n377 = Number To Decimal String(number=w1280) -> (decimal integer string=w1285:string)  [unwired: 1 in]
            n378 = Replace Array Subset(array=w1275, new element=w1285, index (row)=4 ("인덱스 (행)"), index (col)=3 ("비활성화된 인덱스 (열)")) -> (w1284:string[][])
            n379 = Replace Array Subset(array=w1274, new element=w1285, index (row)=4 ("인덱스 (행)"), index (col)=3 ("비활성화된 인덱스 (열)")) -> (w1283:string[][])
            n380 = Replace Array Subset(array=w1273, new element=w1285, index (row)=4 ("인덱스 (행)"), index (col)=3 ("비활성화된 인덱스 (열)")) -> (w1282:string[][])
            n381 = case shown="10..15" w1272 {
              tunnel: [0 13 33 53] -> w1279
              tunnel: w1284 -> [_ w1301 _ _]
              tunnel: w1283 -> [_ _ w1305 _]
              tunnel: w1282 -> [_ _ _ w1309]
              tunnel: [w1297 w1301 w1304 w1308] -> w1278
              tunnel: [w1296 w1300 w1305 w1307] -> w1277
              tunnel: [w1295 w1299 w1303 w1309] -> w1276
              tunnel: w1274 -> [w1296 w1300 _ w1307]
              tunnel: w1273 -> [w1295 w1299 w1303 _]
              tunnel: w1275 -> [w1297 _ w1304 w1308]
              frame 0, Default {
              }
              frame 10..15 {
              }
              frame 30..35 {
              }
              frame 50..55 {
              }
            }
            n382 = Bundle By Name(cluster=w1281, "TX_그래프_LED"=w1292, "TX_그래프2_LED"=w1292, "TX_그래프3_LED"=w1292, "TX_그래프4_LED"=TRUE, "TX_그래프5_LED"=w1292, "유속데이터흐름표_10분"=w1278, "유속데이터흐름표_30분"=w1277, "유속데이터흐름표_50분"=w1276) -> (w1294:T6)
          }
          frame 5 {
            w1313 = FALSE
            n383 = Bundle By Name(cluster=w1312, "TX_그래프_LED"=w1313, "TX_그래프2_LED"=w1313, "TX_그래프3_LED"=w1313, "TX_그래프4_LED"=w1313, "TX_그래프5_LED"=TRUE) -> (w1315:T6)
          }
        }
        n384 = Number To Decimal String(number=w1128) -> (decimal integer string=w1107:string)  [unwired: 1 in]
        n385 = Number To Decimal String(number=w1099) -> (decimal integer string=w1106:string)  [unwired: 1 in]
        n386 = Number To Decimal String(number=w1127) -> (decimal integer string=w1139:string)  [unwired: 1 in]
        n387 = Number To Decimal String(number=w1126) -> (decimal integer string=w1138:string)  [unwired: 1 in]
        n388 = Concatenate Strings("_Q_" ("시간 포맷 문자열 (%c)"), w1139) -> (w1136:string)
        n389 = Concatenate Strings("_Order : " ("시간 포맷 문자열 (%c)"), w1138) -> (w1135:string)
        n390 = Array Subset(array=w1121, index (row)=0 ("인덱스"), length (row)=7 ("길이"), index (col)=0 ("인덱스"), length (col)=1 ("길이")) -> (w1119:string[][])
        n391 = Format Date/Time String(time format string (%c)="%Y_%m_%d_%H_%M_" ("시간 포맷 문자열 (%c)")) -> (date/time string=w1133:string)  [unwired: 2 in]
        n392 = Array Subset(array=w1119, index (row)=3 ("인덱스"), length (row)=2 ("길이")) -> (w1120:string[][])  [unwired: 2 in]
        n393 = Bundle(w1146, w1145) -> (→"Station_5":cluster{dbl[], i32[]})  [unwired: 1 in]
        n394 = for {
          tunnel: w1120 -> [w1317] mode=indexing
          shift-right: [w1316] -> w1105
          shift-left: string[] [] -> [w1318]
          n395 = Build Array (concatenate)(w1318, w1317) -> (w1316:string[])
        }
        n396 = Concatenate Strings(w1132, w1133, w1108, "_Station_" ("시간 포맷 문자열 (%c)"), w1107, "_Station : " ("시간 포맷 문자열 (%c)"), w1106, w1136, w1135, "\r") -> (w1131:string)
        n397 = Format Date/Time String(time format string (%c)="%Y_%m_%d_%H_" ("시간 포맷 문자열 (%c)")) -> (date/time string=w1110:string)  [unwired: 2 in]
        n398 = Number To Decimal String(number=w1103) -> (decimal integer string=w1109:string)  [unwired: 1 in]
        n399 = Concatenate Strings(w1110, w1109) -> (→"Station_5_수신시작시간":string)
        n400 = Bundle By Name(cluster=w1129, "로그기록"=w1131, "RX_그래프_LED"=w1124, "RX_그래프2_LED"=w1124, "RX_그래프3_LED"=w1124, "RX_그래프4_LED"=w1124, "RX_그래프5_LED"=TRUE) -> (w1130:T5)
        n401 = Build Array (concatenate)(w1110, w1109, w1108, w1107, w1106, w1105) -> (w1104:string[])
        n402 = call "Save_teplete(Subvi).vi"("숫자형"=2, "배열"=w1104) -> ()  [unwired: 10 in]
      }
    }
    n403 = Unbundle By Name(w124) -> ("TX_그래프_LED"=→"TX_LED_1":bool, "TX_그래프2_LED"=→"TX_LED_2":bool, "TX_그래프3_LED"=→"TX_LED_3":bool, "TX_그래프4_LED"=→"TX_LED_4":bool, "TX_그래프5_LED"=→"TX_LED_5":bool, "유속데이터흐름표_10분"=w113:string[][], "유속데이터흐름표_30분"=w112:string[][], "유속데이터흐름표_50분"=w111:string[][])
    n404 = Unbundle By Name(w119) -> ("로그기록"=→"데이터 통계 현황_결과창":string, "RX_그래프_LED"=→"RX_LED_1":bool, "RX_그래프2_LED"=→"RX_LED_2":bool, "RX_그래프3_LED"=→"RX_LED_3":bool, "RX_그래프4_LED"=→"RX_LED_4":bool, "RX_그래프5_LED"=→"RX_LED_5":bool)
    n405 = property on="유속 데이터 흐름표_10분" class="MCListbox (엄격한)"("ItemNames"=w113) -> ()  [unwired: 2 in, 2 out]
    n406 = property on="유속 데이터 흐름표_30분" class="MCListbox (엄격한)"("ItemNames"=w112) -> ()  [unwired: 2 in, 2 out]
    n407 = property on="유속 데이터 흐름표_50분" class="MCListbox (엄격한)"("ItemNames"=w111) -> ()  [unwired: 2 in, 2 out]
  }
  n408 = while {
    tunnel: w2 -> [w1348]
    tunnel: w1 -> [w1347]
    tunnel: w19 -> [w1344]
    tunnel: w18 -> [w1343]
    shift-right: [w1336] -> _
    shift-left: string[][] [["", "", "", "", "", ""], ["", "", "", "", "", ""], ["", "", "", "", "", ""], ["", "", "", "", "", ""], ["", "", "", "", "", ""], ["", "", "", "", "", ""], ["", "", "", "", "", ""], ["", "", "", "", "", "0"], ["", "", "", "", "", ""], ["", "", "", "", "", ""], ["", "", "", "", "", ""], ["", "", "", "", "", ""], ["", "", "", "", "", ""]] -> [w1337]
    tunnel: [errorcluster {"status"=FALSE, "code"=0, "source"=""} ("에러 상수")] -> w11
    stop <- w1345 stop-if-true
    # "Number 데이터 분리 후 리스트 박스 열에 데이터 대체"
    # "7 index: Number"
    # "Queue2: BDDATA 처리 LOOP"
    n409 = Dequeue Element(queue=w1348, error in (no error)=w1347) -> (queue out=w1342:refnum<queue>, element=w1346:T9, error out=w1341:errorcluster)  [unwired: 1 in, 1 out]
    n410 = Dequeue Element(queue=w1344, error in (no error)=w1343) -> (element=w1338:string[])  [unwired: 1 in, 3 out]
    n411 = case shown="\"Mqtt_Subscribe\"" w1346 {
      tunnel: [_ _ TRUE] -> w1345
      tunnel: w1342 -> [_ w1386 w1391]
      tunnel: w1341 -> [_ w1385 w1390]
      frame "초기화", Default {
      }
      frame "Mqtt_Subscribe" {
        n412 = Enqueue Element(queue=w1386, element=Brain_Loop_CTL."Mqtt_Subscribe", error in (no error)=w1385) -> ()  [unwired: 1 in, 3 out]
      }
      frame "정지" {
        n413 = Flush Queue(queue=w1391, error in (no error)=w1390) -> (queue out=w1389:refnum<queue>, error out=w1388:errorcluster)  [unwired: 1 out]
        n414 = Enqueue Element(queue=w1389, element=Brain_Loop_CTL."정지", error in (no error)=w1388) -> ()  [unwired: 1 in, 3 out]
      }
    }
    n415 = Index Array(array=w1338, index=7 ("인덱스")) -> (element=w1339:string)
    n416 = case shown="\"1\"" w1339 {
      tunnel: w1338 -> [_ w1353 w1360 w1367 w1374 w1381]
      tunnel: w1337 -> [w1349 w1356 w1363 w1370 w1377 w1384]
      tunnel: [w1349 w1354 w1361 w1368 w1375 w1382] -> w1336
      frame "거짓", Default {
      }
      frame "1" {
        # "Number 데이터 분리 후 리스트 박스 열에 데이처 대체"
        n417 = Array Subset(array=w1353, index=0 ("차원 크기"), length=7 ("차원 크기")) -> (w1350:string[])
        n418 = Replace Array Subset(array=w1356, new element=w1350, index (col)=0 ("비활성화된 인덱스 (열)")) -> (w1354:string[][])  [unwired: 1 in]
        n419 = property on="Station_현황_TRX_Controller" class="MCListbox (엄격한)"("ItemNames"=w1354) -> ()  [unwired: 2 in, 2 out]
      }
      frame "2" {
        n420 = Array Subset(array=w1360, index=0 ("차원 크기"), length=7 ("차원 크기")) -> (w1357:string[])
        n421 = Replace Array Subset(array=w1363, new element=w1357, index (col)=1 ("비활성화된 인덱스 (열)")) -> (w1361:string[][])  [unwired: 1 in]
        n422 = property on="Station_현황_TRX_Controller" class="MCListbox (엄격한)"("ItemNames"=w1361) -> ()  [unwired: 2 in, 2 out]
      }
      frame "3" {
        n423 = Array Subset(array=w1367, index=0 ("차원 크기"), length=7 ("차원 크기")) -> (w1364:string[])
        n424 = Replace Array Subset(array=w1370, new element=w1364, index (col)=2 ("비활성화된 인덱스 (열)")) -> (w1368:string[][])  [unwired: 1 in]
        n425 = property on="Station_현황_TRX_Controller" class="MCListbox (엄격한)"("ItemNames"=w1368) -> ()  [unwired: 2 in, 2 out]
      }
      frame "4" {
        n426 = Array Subset(array=w1374, index=0 ("차원 크기"), length=7 ("차원 크기")) -> (w1371:string[])
        n427 = Replace Array Subset(array=w1377, new element=w1371, index (col)=3 ("비활성화된 인덱스 (열)")) -> (w1375:string[][])  [unwired: 1 in]
        n428 = property on="Station_현황_TRX_Controller" class="MCListbox (엄격한)"("ItemNames"=w1375) -> ()  [unwired: 2 in, 2 out]
      }
      frame "5" {
        n429 = Array Subset(array=w1381, index=0 ("차원 크기"), length=7 ("차원 크기")) -> (w1378:string[])
        n430 = Replace Array Subset(array=w1384, new element=w1378, index (col)=4 ("비활성화된 인덱스 (열)")) -> (w1382:string[][])  [unwired: 1 in]
        n431 = property on="Station_현황_TRX_Controller" class="MCListbox (엄격한)"("ItemNames"=w1382) -> ()  [unwired: 2 in, 2 out]
      }
    }
  }
  n432 = while {
    tunnel: w2 -> [w1399]
    tunnel: w1 -> [w1398]
    stop <- w1397 stop-if-true
    n433 = Dequeue Element(queue=w1399, error in (no error)=w1398) -> (queue out=w1401:refnum<queue>, element=w1400:T9, error out=w1402:errorcluster)  [unwired: 1 in, 1 out]
    n434 = case shown="\"Mqtt_Subscribe\"" w1400 {
      tunnel: [_ _ TRUE] -> w1397
      tunnel: w1401 -> [_ w1682 w1687]
      tunnel: w1402 -> [_ w1681 w1686]
      frame "초기화", Default {
      }
      frame "Mqtt_Subscribe" {
        n435 = Enqueue Element(queue=w1682, element=Brain_Loop_CTL."Mqtt_Subscribe", error in (no error)=w1681) -> ()  [unwired: 1 in, 3 out]
      }
      frame "정지" {
        n436 = Flush Queue(queue=w1687, error in (no error)=w1686) -> (queue out=w1685:refnum<queue>, error out=w1684:errorcluster)  [unwired: 1 out]
        n437 = Enqueue Element(queue=w1685, element=Brain_Loop_CTL."정지", error in (no error)=w1684) -> ()  [unwired: 1 in, 3 out]
      }
    }
    n438 = Format Date/Time String(time format string (%c)="%M" ("시간 포맷 문자열 (%c)")) -> (date/time string=w1396:string)  [unwired: 2 in]
    n439 = Decimal String To Number(string=w1396) -> ()  [unwired: 2 in, 2 out]
    n440 = case shown="56" "숫자형" {
      frame 0, Default {
      }
      frame 16 {
        w1416 = 0 ("인덱스 (행)")
        w1413 = 0 ("인덱스 (행)")
        w1422 = 0 ("인덱스 (행)")
        w1425 = 0 ("인덱스 (행)")
        w1442 = 0 ("인덱스 (행)")
        w1439 = 0 ("인덱스 (행)")
        w1448 = 0 ("인덱스 (행)")
        w1451 = 0 ("인덱스 (행)")
        w1468 = 0 ("인덱스 (행)")
        w1465 = 0 ("인덱스 (행)")
        w1474 = 0 ("인덱스 (행)")
        w1477 = 0 ("인덱스 (행)")
        w1494 = 0 ("인덱스 (행)")
        w1491 = 0 ("인덱스 (행)")
        w1500 = 0 ("인덱스 (행)")
        w1503 = 0 ("인덱스 (행)")
        w1520 = 0 ("인덱스 (행)")
        w1517 = 0 ("인덱스 (행)")
        w1526 = 0 ("인덱스 (행)")
        w1529 = 0 ("인덱스 (행)")
        w1406 = 1 ("길이")
        n441 = property on="유속 데이터 흐름표_10분" class="MCListbox (엄격한)"() -> ("ItemNames"=w1407:string[][])  [unwired: 2 in, 2 out]
        n442 = property on="Station_현황_GPS" class="MCListbox (엄격한)"() -> ("ItemNames"=w1535:string[][])  [unwired: 2 in, 2 out]
        n443 = call "Result_distance_GPS(Subvi).vi"("아이템 이름"=w1535) -> ("1_2_distance[m]"=w1522:dbl, "1_3_distance[m]"=w1509:dbl, "1_4_distance[m]"=w1496:dbl, "1_5_distance[m]"=w1483:dbl, "2_3_distance[m]"=w1470:dbl, "2_4_distance[m]"=w1457:dbl, "2_5_distance[m]"=w1444:dbl, "4_5_distance[m]"=w1403:dbl, "3_5_distance[m]"=w1418:dbl, "3_4_distance[m]"=w1431:dbl)  [unwired: 5 in]
        n444 = Array Subset(array=w1407, index (row)=1 ("인덱스"), length (row)=w1406, index (col)=0 ("인덱스"), length (col)=w1406) -> (w1530:string[][])
        n445 = Array Subset(array=w1407, index (row)=4 ("인덱스"), length (row)=w1406, index (col)=0 ("인덱스"), length (col)=w1406) -> (w1490:string[][])
        n446 = Array Subset(array=w1407, index (row)=3 ("인덱스"), length (row)=w1406, index (col)=1 ("인덱스"), length (col)=w1406) -> (w1464:string[][])
        n447 = Array Subset(array=w1407, index (row)=0 ("인덱스"), length (row)=w1406, index (col)=1 ("인덱스"), length (col)=w1406) -> (w1525:string[][])
        n448 = Array Subset(array=w1407, index (row)=2 ("인덱스"), length (row)=w1406, index (col)=0 ("인덱스"), length (col)=w1406) -> (w1516:string[][])
        n449 = Array Subset(array=w1407, index (row)=3 ("인덱스"), length (row)=w1406, index (col)=0 ("인덱스"), length (col)=w1406) -> (w1504:string[][])
        n450 = Array Subset(array=w1407, index (row)=0 ("인덱스"), length (row)=w1406, index (col)=4 ("인덱스"), length (col)=w1406) -> (w1495:string[][])
        n451 = Array Subset(array=w1407, index (row)=2 ("인덱스"), length (row)=w1406, index (col)=1 ("인덱스"), length (col)=w1406) -> (w1478:string[][])
        n452 = Array Subset(array=w1407, index (row)=1 ("인덱스"), length (row)=w1406, index (col)=3 ("인덱스"), length (col)=w1406) -> (w1469:string[][])
        n453 = Array Subset(array=w1407, index (row)=4 ("인덱스"), length (row)=w1406, index (col)=1 ("인덱스"), length (col)=w1406) -> (w1452:string[][])
        n454 = Array Subset(array=w1407, index (row)=0 ("인덱스"), length (row)=w1406, index (col)=2 ("인덱스"), length (col)=w1406) -> (w1521:string[][])
        n455 = Array Subset(array=w1407, index (row)=0 ("인덱스"), length (row)=w1406, index (col)=3 ("인덱스"), length (col)=w1406) -> (w1499:string[][])
        n456 = Array Subset(array=w1407, index (row)=1 ("인덱스"), length (row)=w1406, index (col)=2 ("인덱스"), length (col)=w1406) -> (w1473:string[][])
        n457 = Array Subset(array=w1407, index (row)=1 ("인덱스"), length (row)=w1406, index (col)=4 ("인덱스"), length (col)=w1406) -> (w1447:string[][])
        n458 = Array Subset(array=w1407, index (row)=4 ("인덱스"), length (row)=w1406, index (col)=3 ("인덱스"), length (col)=w1406) -> (w1412:string[][])
        n459 = Array Subset(array=w1407, index (row)=3 ("인덱스"), length (row)=w1406, index (col)=2 ("인덱스"), length (col)=w1406) -> (w1438:string[][])
        n460 = Array Subset(array=w1407, index (row)=4 ("인덱스"), length (row)=w1406, index (col)=2 ("인덱스"), length (col)=w1406) -> (w1426:string[][])
        n461 = Array Subset(array=w1407, index (row)=3 ("인덱스"), length (row)=w1406, index (col)=4 ("인덱스"), length (col)=w1406) -> (w1417:string[][])
        n462 = Array Subset(array=w1407, index (row)=2 ("인덱스"), length (row)=w1406, index (col)=3 ("인덱스"), length (col)=w1406) -> (w1443:string[][])
        n463 = Array Subset(array=w1407, index (row)=2 ("인덱스"), length (row)=w1406, index (col)=4 ("인덱스"), length (col)=w1406) -> (w1421:string[][])
        n464 = Index Array(array=w1530, index (row)=w1529, index (col)=w1529) -> (element=w1528:string)
        n465 = Index Array(array=w1525, index (row)=w1526, index (col)=w1526) -> (element=w1527:string)
        n466 = Index Array(array=w1490, index (row)=w1491, index (col)=w1491) -> (element=w1492:string)
        n467 = Index Array(array=w1495, index (row)=w1494, index (col)=w1494) -> (element=w1493:string)
        n468 = Index Array(array=w1464, index (row)=w1465, index (col)=w1465) -> (element=w1466:string)
        n469 = Index Array(array=w1469, index (row)=w1468, index (col)=w1468) -> (element=w1467:string)
        n470 = Index Array(array=w1516, index (row)=w1517, index (col)=w1517) -> (element=w1518:string)
        n471 = Index Array(array=w1521, index (row)=w1520, index (col)=w1520) -> (element=w1519:string)
        n472 = Index Array(array=w1504, index (row)=w1503, index (col)=w1503) -> (element=w1502:string)
        n473 = Index Array(array=w1499, index (row)=w1500, index (col)=w1500) -> (element=w1501:string)
        n474 = Index Array(array=w1478, index (row)=w1477, index (col)=w1477) -> (element=w1476:string)
        n475 = Index Array(array=w1473, index (row)=w1474, index (col)=w1474) -> (element=w1475:string)
        n476 = Index Array(array=w1452, index (row)=w1451, index (col)=w1451) -> (element=w1450:string)
        n477 = Index Array(array=w1447, index (row)=w1448, index (col)=w1448) -> (element=w1449:string)
        n478 = Index Array(array=w1412, index (row)=w1413, index (col)=w1413) -> (element=w1414:string)
        n479 = Index Array(array=w1417, index (row)=w1416, index (col)=w1416) -> (element=w1415:string)
        n480 = Index Array(array=w1438, index (row)=w1439, index (col)=w1439) -> (element=w1440:string)
        n481 = Index Array(array=w1443, index (row)=w1442, index (col)=w1442) -> (element=w1441:string)
        n482 = Index Array(array=w1426, index (row)=w1425, index (col)=w1425) -> (element=w1424:string)
        n483 = Index Array(array=w1421, index (row)=w1422, index (col)=w1422) -> (element=w1423:string)
        n484 = Decimal String To Number(string=w1528) -> (number=w1524:i32)  [unwired: 2 in, 1 out]
        n485 = Decimal String To Number(string=w1527) -> (number=w1523:i32)  [unwired: 2 in, 1 out]
        n486 = Decimal String To Number(string=w1492) -> (number=w1485:i32)  [unwired: 2 in, 1 out]
        n487 = Decimal String To Number(string=w1493) -> (number=w1484:i32)  [unwired: 2 in, 1 out]
        n488 = Decimal String To Number(string=w1466) -> (number=w1459:i32)  [unwired: 2 in, 1 out]
        n489 = Decimal String To Number(string=w1467) -> (number=w1458:i32)  [unwired: 2 in, 1 out]
        n490 = Decimal String To Number(string=w1518) -> (number=w1511:i32)  [unwired: 2 in, 1 out]
        n491 = Decimal String To Number(string=w1519) -> (number=w1510:i32)  [unwired: 2 in, 1 out]
        n492 = Decimal String To Number(string=w1502) -> (number=w1498:i32)  [unwired: 2 in, 1 out]
        n493 = Decimal String To Number(string=w1501) -> (number=w1497:i32)  [unwired: 2 in, 1 out]
        n494 = Decimal String To Number(string=w1476) -> (number=w1472:i32)  [unwired: 2 in, 1 out]
        n495 = Decimal String To Number(string=w1475) -> (number=w1471:i32)  [unwired: 2 in, 1 out]
        n496 = Decimal String To Number(string=w1450) -> (number=w1446:i32)  [unwired: 2 in, 1 out]
        n497 = Decimal String To Number(string=w1449) -> (number=w1445:i32)  [unwired: 2 in, 1 out]
        n498 = Decimal String To Number(string=w1414) -> (number=w1405:i32)  [unwired: 2 in, 1 out]
        n499 = Decimal String To Number(string=w1415) -> (number=w1404:i32)  [unwired: 2 in, 1 out]
        n500 = Decimal String To Number(string=w1440) -> (number=w1433:i32)  [unwired: 2 in, 1 out]
        n501 = Decimal String To Number(string=w1441) -> (number=w1432:i32)  [unwired: 2 in, 1 out]
        n502 = Decimal String To Number(string=w1424) -> (number=w1420:i32)  [unwired: 2 in, 1 out]
        n503 = Decimal String To Number(string=w1423) -> (number=w1419:i32)  [unwired: 2 in, 1 out]
        n504 = call "Col_Velocity(Subvi).vi"("거리"=w1522, "Station_index_2"=w1523, "Station_index_1"=w1524) -> ()  [unwired: 7 in, 2 out]
        n505 = call "Col_Velocity(Subvi).vi"("거리"=w1509, "Station_index_2"=w1510, "Station_index_1"=w1511) -> ()  [unwired: 7 in, 2 out]
        n506 = call "Col_Velocity(Subvi).vi"("거리"=w1496, "Station_index_2"=w1497, "Station_index_1"=w1498) -> ()  [unwired: 7 in, 2 out]
        n507 = call "Col_Velocity(Subvi).vi"("거리"=w1483, "Station_index_2"=w1484, "Station_index_1"=w1485) -> ()  [unwired: 7 in, 2 out]
        n508 = call "Col_Velocity(Subvi).vi"("거리"=w1470, "Station_index_2"=w1471, "Station_index_1"=w1472) -> ()  [unwired: 7 in, 2 out]
        n509 = call "Col_Velocity(Subvi).vi"("거리"=w1457, "Station_index_2"=w1458, "Station_index_1"=w1459) -> ()  [unwired: 7 in, 2 out]
        n510 = call "Col_Velocity(Subvi).vi"("거리"=w1444, "Station_index_2"=w1445, "Station_index_1"=w1446) -> ()  [unwired: 7 in, 2 out]
        n511 = call "Col_Velocity(Subvi).vi"("거리"=w1431, "Station_index_2"=w1432, "Station_index_1"=w1433) -> ()  [unwired: 7 in, 2 out]
        n512 = call "Col_Velocity(Subvi).vi"("거리"=w1418, "Station_index_2"=w1419, "Station_index_1"=w1420) -> ()  [unwired: 7 in, 2 out]
        n513 = call "Col_Velocity(Subvi).vi"("거리"=w1403, "Station_index_2"=w1404, "Station_index_1"=w1405) -> ()  [unwired: 7 in, 2 out]
      }
      frame 36 {
        w1549 = 0 ("인덱스 (행)")
        w1546 = 0 ("인덱스 (행)")
        w1555 = 0 ("인덱스 (행)")
        w1558 = 0 ("인덱스 (행)")
        w1575 = 0 ("인덱스 (행)")
        w1572 = 0 ("인덱스 (행)")
        w1581 = 0 ("인덱스 (행)")
        w1584 = 0 ("인덱스 (행)")
        w1601 = 0 ("인덱스 (행)")
        w1598 = 0 ("인덱스 (행)")
        w1607 = 0 ("인덱스 (행)")
        w1610 = 0 ("인덱스 (행)")
        w1627 = 0 ("인덱스 (행)")
        w1624 = 0 ("인덱스 (행)")
        w1633 = 0 ("인덱스 (행)")
        w1636 = 0 ("인덱스 (행)")
        w1653 = 0 ("인덱스 (행)")
        w1650 = 0 ("인덱스 (행)")
        w1659 = 0 ("인덱스 (행)")
        w1662 = 0 ("인덱스 (행)")
        w1540 = 1 ("길이")
        n514 = property on="Station_현황_GPS" class="MCListbox (엄격한)"() -> ("ItemNames"=w1668:string[][])  [unwired: 2 in, 2 out]
        n515 = property on="유속 데이터 흐름표_30분" class="MCListbox (엄격한)"() -> ("ItemNames"=w1536:string[][])  [unwired: 2 in, 2 out]
        n516 = call "Result_distance_GPS(Subvi).vi"("아이템 이름"=w1668) -> ("1_2_distance[m]"=w1655:dbl, "1_3_distance[m]"=w1642:dbl, "1_4_distance[m]"=w1629:dbl, "1_5_distance[m]"=w1616:dbl, "2_3_distance[m]"=w1603:dbl, "2_4_distance[m]"=w1590:dbl, "2_5_distance[m]"=w1577:dbl, "4_5_distance[m]"=w1537:dbl, "3_5_distance[m]"=w1551:dbl, "3_4_distance[m]"=w1564:dbl)  [unwired: 5 in]
        n517 = Array Subset(array=w1536, index (row)=1 ("인덱스"), length (row)=w1540, index (col)=0 ("인덱스"), length (col)=w1540) -> (w1663:string[][])
        n518 = Array Subset(array=w1536, index (row)=4 ("인덱스"), length (row)=w1540, index (col)=0 ("인덱스"), length (col)=w1540) -> (w1623:string[][])
        n519 = Array Subset(array=w1536, index (row)=3 ("인덱스"), length (row)=w1540, index (col)=1 ("인덱스"), length (col)=w1540) -> (w1597:string[][])
        n520 = Array Subset(array=w1536, index (row)=0 ("인덱스"), length (row)=w1540, index (col)=1 ("인덱스"), length (col)=w1540) -> (w1658:string[][])
        n521 = Array Subset(array=w1536, index (row)=2 ("인덱스"), length (row)=w1540, index (col)=0 ("인덱스"), length (col)=w1540) -> (w1649:string[][])
        n522 = Array Subset(array=w1536, index (row)=3 ("인덱스"), length (row)=w1540, index (col)=0 ("인덱스"), length (col)=w1540) -> (w1637:string[][])
        n523 = Array Subset(array=w1536, index (row)=0 ("인덱스"), length (row)=w1540, index (col)=4 ("인덱스"), length (col)=w1540) -> (w1628:string[][])
        n524 = Array Subset(array=w1536, index (row)=2 ("인덱스"), length (row)=w1540, index (col)=1 ("인덱스"), length (col)=w1540) -> (w1611:string[][])
        n525 = Array Subset(array=w1536, index (row)=1 ("인덱스"), length (row)=w1540, index (col)=3 ("인덱스"), length (col)=w1540) -> (w1602:string[][])
        n526 = Array Subset(array=w1536, index (row)=4 ("인덱스"), length (row)=w1540, index (col)=1 ("인덱스"), length (col)=w1540) -> (w1585:string[][])
        n527 = Array Subset(array=w1536, index (row)=0 ("인덱스"), length (row)=w1540, index (col)=2 ("인덱스"), length (col)=w1540) -> (w1654:string[][])
        n528 = Array Subset(array=w1536, index (row)=0 ("인덱스"), length (row)=w1540, index (col)=3 ("인덱스"), length (col)=w1540) -> (w1632:string[][])
        n529 = Array Subset(array=w1536, index (row)=1 ("인덱스"), length (row)=w1540, index (col)=2 ("인덱스"), length (col)=w1540) -> (w1606:string[][])
        n530 = Array Subset(array=w1536, index (row)=1 ("인덱스"), length (row)=w1540, index (col)=4 ("인덱스"), length (col)=w1540) -> (w1580:string[][])
        n531 = Array Subset(array=w1536, index (row)=4 ("인덱스"), length (row)=w1540, index (col)=3 ("인덱스"), length (col)=w1540) -> (w1545:string[][])
        n532 = Array Subset(array=w1536, index (row)=3 ("인덱스"), length (row)=w1540, index (col)=2 ("인덱스"), length (col)=w1540) -> (w1571:string[][])
        n533 = Array Subset(array=w1536, index (row)=4 ("인덱스"), length (row)=w1540, index (col)=2 ("인덱스"), length (col)=w1540) -> (w1559:string[][])
        n534 = Array Subset(array=w1536, index (row)=3 ("인덱스"), length (row)=w1540, index (col)=4 ("인덱스"), length (col)=w1540) -> (w1550:string[][])
        n535 = Array Subset(array=w1536, index (row)=2 ("인덱스"), length (row)=w1540, index (col)=3 ("인덱스"), length (col)=w1540) -> (w1576:string[][])
        n536 = Array Subset(array=w1536, index (row)=2 ("인덱스"), length (row)=w1540, index (col)=4 ("인덱스"), length (col)=w1540) -> (w1554:string[][])
        n537 = Index Array(array=w1663, index (row)=w1662, index (col)=w1662) -> (element=w1661:string)
        n538 = Index Array(array=w1658, index (row)=w1659, index (col)=w1659) -> (element=w1660:string)
        n539 = Index Array(array=w1623, index (row)=w1624, index (col)=w1624) -> (element=w1625:string)
        n540 = Index Array(array=w1628, index (row)=w1627, index (col)=w1627) -> (element=w1626:string)
        n541 = Index Array(array=w1597, index (row)=w1598, index (col)=w1598) -> (element=w1599:string)
        n542 = Index Array(array=w1602, index (row)=w1601, index (col)=w1601) -> (element=w1600:string)
        n543 = Index Array(array=w1649, index (row)=w1650, index (col)=w1650) -> (element=w1651:string)
        n544 = Index Array(array=w1654, index (row)=w1653, index (col)=w1653) -> (element=w1652:string)
        n545 = Index Array(array=w1637, index (row)=w1636, index (col)=w1636) -> (element=w1635:string)
        n546 = Index Array(array=w1632, index (row)=w1633, index (col)=w1633) -> (element=w1634:string)
        n547 = Index Array(array=w1611, index (row)=w1610, index (col)=w1610) -> (element=w1609:string)
        n548 = Index Array(array=w1606, index (row)=w1607, index (col)=w1607) -> (element=w1608:string)
        n549 = Index Array(array=w1585, index (row)=w1584, index (col)=w1584) -> (element=w1583:string)
        n550 = Index Array(array=w1580, index (row)=w1581, index (col)=w1581) -> (element=w1582:string)
        n551 = Index Array(array=w1545, index (row)=w1546, index (col)=w1546) -> (element=w1547:string)
        n552 = Index Array(array=w1550, index (row)=w1549, index (col)=w1549) -> (element=w1548:string)
        n553 = Index Array(array=w1571, index (row)=w1572, index (col)=w1572) -> (element=w1573:string)
        n554 = Index Array(array=w1576, index (row)=w1575, index (col)=w1575) -> (element=w1574:string)
        n555 = Index Array(array=w1559, index (row)=w1558, index (col)=w1558) -> (element=w1557:string)
        n556 = Index Array(array=w1554, index (row)=w1555, index (col)=w1555) -> (element=w1556:string)
        n557 = Decimal String To Number(string=w1661) -> (number=w1657:i32)  [unwired: 2 in, 1 out]
        n558 = Decimal String To Number(string=w1660) -> (number=w1656:i32)  [unwired: 2 in, 1 out]
        n559 = Decimal String To Number(string=w1625) -> (number=w1618:i32)  [unwired: 2 in, 1 out]
        n560 = Decimal String To Number(string=w1626) -> (number=w1617:i32)  [unwired: 2 in, 1 out]
        n561 = Decimal String To Number(string=w1599) -> (number=w1592:i32)  [unwired: 2 in, 1 out]
        n562 = Decimal String To Number(string=w1600) -> (number=w1591:i32)  [unwired: 2 in, 1 out]
        n563 = Decimal String To Number(string=w1651) -> (number=w1644:i32)  [unwired: 2 in, 1 out]
        n564 = Decimal String To Number(string=w1652) -> (number=w1643:i32)  [unwired: 2 in, 1 out]
        n565 = Decimal String To Number(string=w1635) -> (number=w1631:i32)  [unwired: 2 in, 1 out]
        n566 = Decimal String To Number(string=w1634) -> (number=w1630:i32)  [unwired: 2 in, 1 out]
        n567 = Decimal String To Number(string=w1609) -> (number=w1605:i32)  [unwired: 2 in, 1 out]
        n568 = Decimal String To Number(string=w1608) -> (number=w1604:i32)  [unwired: 2 in, 1 out]
        n569 = Decimal String To Number(string=w1583) -> (number=w1579:i32)  [unwired: 2 in, 1 out]
        n570 = Decimal String To Number(string=w1582) -> (number=w1578:i32)  [unwired: 2 in, 1 out]
        n571 = Decimal String To Number(string=w1547) -> (number=w1539:i32)  [unwired: 2 in, 1 out]
        n572 = Decimal String To Number(string=w1548) -> (number=w1538:i32)  [unwired: 2 in, 1 out]
        n573 = Decimal String To Number(string=w1573) -> (number=w1566:i32)  [unwired: 2 in, 1 out]
        n574 = Decimal String To Number(string=w1574) -> (number=w1565:i32)  [unwired: 2 in, 1 out]
        n575 = Decimal String To Number(string=w1557) -> (number=w1553:i32)  [unwired: 2 in, 1 out]
        n576 = Decimal String To Number(string=w1556) -> (number=w1552:i32)  [unwired: 2 in, 1 out]
        n577 = call "Col_Velocity(Subvi).vi"("거리"=w1655, "Station_index_2"=w1656, "Station_index_1"=w1657) -> ()  [unwired: 7 in, 2 out]
        n578 = call "Col_Velocity(Subvi).vi"("거리"=w1642, "Station_index_2"=w1643, "Station_index_1"=w1644) -> ()  [unwired: 7 in, 2 out]
        n579 = call "Col_Velocity(Subvi).vi"("거리"=w1629, "Station_index_2"=w1630, "Station_index_1"=w1631) -> ()  [unwired: 7 in, 2 out]
        n580 = call "Col_Velocity(Subvi).vi"("거리"=w1616, "Station_index_2"=w1617, "Station_index_1"=w1618) -> ()  [unwired: 7 in, 2 out]
        n581 = call "Col_Velocity(Subvi).vi"("거리"=w1603, "Station_index_2"=w1604, "Station_index_1"=w1605) -> ()  [unwired: 7 in, 2 out]
        n582 = call "Col_Velocity(Subvi).vi"("거리"=w1590, "Station_index_2"=w1591, "Station_index_1"=w1592) -> ()  [unwired: 7 in, 2 out]
        n583 = call "Col_Velocity(Subvi).vi"("거리"=w1577, "Station_index_2"=w1578, "Station_index_1"=w1579) -> ()  [unwired: 7 in, 2 out]
        n584 = call "Col_Velocity(Subvi).vi"("거리"=w1564, "Station_index_2"=w1565, "Station_index_1"=w1566) -> ()  [unwired: 7 in, 2 out]
        n585 = call "Col_Velocity(Subvi).vi"("거리"=w1551, "Station_index_2"=w1552, "Station_index_1"=w1553) -> ()  [unwired: 7 in, 2 out]
        n586 = call "Col_Velocity(Subvi).vi"("거리"=w1537, "Station_index_2"=w1538, "Station_index_1"=w1539) -> ()  [unwired: 7 in, 2 out]
      }
      frame 56 {
        n587 = property on="유속 데이터 흐름표_50분" class="MCListbox (엄격한)"() -> ("ItemNames"=w1679:string[][])  [unwired: 2 in, 2 out]
        n588 = property on="Station_현황_GPS" class="MCListbox (엄격한)"() -> ("ItemNames"=w1680:string[][])  [unwired: 2 in, 2 out]
        n589 = call "Graph_Water_Velocity(Subvi).vi"("ItemNames 2"=w1680, "ItemNames"=w1679) -> ("Water_Velocity"=→"Water_Velocity":dbl, "Water_Velocity 2"=→"Water_Velocity 2":dbl, "Water_Velocity 10"=→"Water_Velocity 10":dbl, "Water_Velocity 3"=→"Water_Velocity 3":dbl, "Water_Velocity 9"=→"Water_Velocity 9":dbl, "Water_Velocity 4"=→"Water_Velocity 4":dbl, "Water_Velocity 8"=→"Water_Velocity 8":dbl, "Water_Velocity 7"=→"Water_Velocity 7":dbl, "Water_Velocity 6"=→"Water_Velocity 6":dbl, "Water_Velocity 5"=→"Water_Velocity 5":dbl)  [unwired: 4 in]
      }
    }
  }
  n590 = while {
    tunnel: w25 -> [w1700]
    tunnel: w15 -> [w1699]
    tunnel: [errorcluster {"status"=FALSE, "code"=0, "source"=""} ("에러 상수")] -> w22
    tunnel: w2 -> [w1693]
    tunnel: w1 -> [w1692]
    shift-right: [w1690] -> _
    shift-left: T7 {"Python 경로"=path "", "Publish 모듈 경로"=path "", "지도 모듈 경로"=path ""} -> [w1691]
    stop <- w1696 stop-if-true
    # "Brain_Loop"
    n591 = Dequeue Element(queue=w1699, error in (no error)=w1700) -> (queue out=w1695:refnum<queue>, element=w1697:T9, error out=w1694:errorcluster)  [unwired: 1 in, 1 out]
    n592 = case shown="\"초기화\", 기본" w1697 {
      tunnel: [_ _ _ _ _ _ _ w1813] -> w1696
      tunnel: w1695 -> [_ _ _ _ _ _ _ _]
      tunnel: w1694 -> [_ _ _ _ _ _ _ _]
      tunnel: w1693 -> [w1718 _ _ _ _ _ _ w1816]
      tunnel: w1692 -> [w1717 _ _ _ _ _ _ w1815]
      tunnel: w1691 -> [w1709 w1720 w1735 w1748 w1806 w1808 w1810 w1812]
      tunnel: [w1708 w1720 w1735 w1748 w1806 w1808 w1810 w1812] -> w1690
      frame "초기화", Default {
        w1702 = FALSE
        w1703 = cluster{dbl[], i32[]} {[], []} ("값(신호)")
        w1713 = string[] ["TMC_SET_1", "TMC_SET_2", "TMC_SET_3", "TMC_SET_4", "TMC_SET_5"]
        # "배터리 전원, 소모전류, 컨트롤 온도, 수온, 압력, Roll, Pitch"
        # "※ 1) GUI가 실행 될때는 (0,0)에서 실행된다. 2) 탭 컨트롤은 데이터 통계로 초기화 한다. 3) 웨이브폼 그래프 값 초기화 4) Station_현황_GPS, TRX_Controller의 리스트 초기화(Brain_LOOP)"
        n593 = Enqueue Element(queue=w1718, element=Brain_Loop_CTL."Mqtt_Subscribe", error in (no error)=w1717) -> ()  [unwired: 1 in, 3 out]
        n594 = Bundle By Name(cluster=w1709, "Python 경로"="Python 경로", "Publish 모듈 경로"="Publish_모듈 경로", "지도 모듈 경로"="지도 모듈 경로") -> (w1708:T7)
        n595 = local write "데이터 통계 현황_결과창"("") -> ()
        n596 = property on="구획" class="Pane"("Origin"=T10 {"Horizontal"=0, "Vertical"=0} ("원점")) -> ()  [unwired: 2 in, 2 out]
        n597 = property on="Station_현황_TRX_Controller" class="MCListbox (엄격한)"("ColHdrString"=w1713, "ItemNames"=string[][] [["", "", "", "", "", "", ""], ["", "", "", "", "", "", ""], ["", "", "", "", "", "", ""], ["", "", "", "", "", "", ""], ["", "", "", "", "", "", ""], ["", "", "", "", "", "", ""], ["", "", "", "", "", "", ""], ["", "", "", "", "", "0", ""], ["", "", "", "", "", "", ""], ["", "", "", "", "", "", ""], ["", "", "", "", "", "", ""], ["", "", "", "", "", "", ""], ["", "", "", "", "", "", ""], ["", "", "", "", "", "", ""]], "RowHdrs[]"=string[] ["배터리 전원", "소모전류", "수온", "압력", "ROLL", "PITCH", "컨트롤 온도", "", ""]) -> ()  [unwired: 2 in, 2 out]
        n598 = property on="Station_현황_GPS" class="MCListbox (엄격한)"("ColHdrString"=w1713, "ItemNames"=string[][] [["", "", "", "", "", ""], ["", "", "", "", "", ""], ["", "", "", "", "", ""], ["", "", "", "", "", ""], ["", "", "", "", "", ""], ["", "", "", "", "", ""], ["", "", "", "", "", ""], ["", "", "", "", "", "0"]], "RowHdrs[]"=string[] ["1PPS", "Latitude", "Longitude"]) -> ()  [unwired: 2 in, 2 out]
        n599 = property on="전체메뉴_탭_컨트롤" class="TabCtl (엄격한)"("Value"=enum32{"지도", "데이터 통계", "관리자", "유속 데이터"}."데이터 통계" ("전체메뉴_탭_컨트롤")) -> ()  [unwired: 2 in, 2 out]
        n600 = call "Save_teplete(Subvi).vi"("숫자형"=1) -> ()  [unwired: 11 in]
        n601 = local write "TX_LED_5"(w1702) -> ()
        n602 = local write "TX_LED_4"(w1702) -> ()
        n603 = local write "TX_LED_3"(w1702) -> ()
        n604 = local write "TX_LED_1"(w1702) -> ()
        n605 = local write "TX_LED_2"(w1702) -> ()
        n606 = local write "RX_LED_5"(w1702) -> ()
        n607 = local write "RX_LED_4"(w1702) -> ()
        n608 = local write "RX_LED_3"(w1702) -> ()
        n609 = local write "RX_LED_2"(w1702) -> ()
        n610 = local write "RX_LED_1"(w1702) -> ()
        n611 = property on="Station_1" class="XYGraph (엄격한)"("Val(Sgnl)"=w1703) -> ()  [unwired: 2 in, 2 out]
        n612 = property on="Station_2" class="XYGraph (엄격한)"("Val(Sgnl)"=w1703) -> ()  [unwired: 2 in, 2 out]
        n613 = property on="Station_3" class="XYGraph (엄격한)"("Val(Sgnl)"=w1703) -> ()  [unwired: 2 in, 2 out]
        n614 = property on="Station_4" class="XYGraph (엄격한)"("Val(Sgnl)"=w1703) -> ()  [unwired: 2 in, 2 out]
        n615 = property on="Station_5" class="XYGraph (엄격한)"("Val(Sgnl)"=w1703) -> ()  [unwired: 2 in, 2 out]
      }
      frame "Mqtt_Publish" {
        # "※ 적용 버튼을 클릭시 Brain_Loop에서 Mqtt_Publish Python 모듈 실행(Brain_LOOP)['Stop,Order,Q,'Start']"
        n616 = Unbundle By Name(w1720) -> ("Python 경로"=w1722:path, "Publish 모듈 경로"=w1721:path)
        n617 = Open Python Session(python version="3.9" ("Python 버전"), python path=w1722) -> (session out=w1731:refnum<k35>, error out=w1727:errorcluster)  [unwired: 1 in]
        n618 = node(w1731, w1721, "Mqtt_Publish" ("함수 이름"), w1727, " ", "Order", "Q 값") -> (w1729:refnum<k35>, w1730:errorcluster)  [unwired: 3 in, 2 out]
        n619 = Close Python Session(session in=w1729, error in=w1730) -> ()  [unwired: 1 out]
        n620 = flat-sequence {
          frame #0 {
            n621 = property on="적용_LED" class="Bool (엄격한)"("Blinking"=TRUE ("점멸")) -> ()  [unwired: 2 in, 2 out]
            n622 = Wait (ms)(milliseconds to wait=u32 2000 ("대기 시간 (ms)")) -> ()  [unwired: 1 out]
          }
          frame #1 {
            n623 = property on="적용_LED" class="Bool (엄격한)"("Blinking"=FALSE ("점멸")) -> ()  [unwired: 2 in, 2 out]
          }
        }
      }
      frame "Mqtt_Publish_2" {
        # "※ 적용 버튼을 클릭시 Brain_Loop에서 Mqtt_Publish Python 모듈 실행(Brain_LOOP)['Stop,Order,Q,'Start']"
        n624 = Unbundle By Name(w1735) -> ("Python 경로"=w1737:path, "Publish 모듈 경로"=w1736:path)
        n625 = Open Python Session(python version="3.9" ("Python 버전"), python path=w1737) -> (session out=w1744:refnum<k35>, error out=w1740:errorcluster)  [unwired: 1 in]
        n626 = node(w1744, w1736, "Mqtt_Publish_2" ("함수 이름"), w1740, " ") -> (w1742:refnum<k35>, w1743:errorcluster)  [unwired: 1 in, 2 out]
        n627 = Close Python Session(session in=w1742, error in=w1743) -> ()  [unwired: 1 out]
        n628 = flat-sequence {
          frame #0 {
            n629 = property on="적용_LED 2" class="Bool (엄격한)"("Blinking"=TRUE ("점멸")) -> ()  [unwired: 2 in, 2 out]
            n630 = Wait (ms)(milliseconds to wait=u32 2000 ("대기 시간 (ms)")) -> ()  [unwired: 1 out]
          }
          frame #1 {
            n631 = property on="적용_LED 2" class="Bool (엄격한)"("Blinking"=FALSE ("점멸")) -> ()  [unwired: 2 in, 2 out]
          }
        }
      }
      frame "지도" {
        # "※ 리스트에 표시된 데이터를 이용하여 Python 모듈과 연동하여 지도 모듈 구현(Brain_LOOP)"
        n632 = property on="Station_현황_GPS" class="MCListbox (엄격한)"() -> ("ItemNames"=w1760:string[][])  [unwired: 2 in, 2 out]
        n633 = Delete From Array(array=w1760, index (row)=2 ("인덱스 (행)")) -> (deleted portion=w1761:string[])  [unwired: 2 in, 1 out]
        n634 = Delete From Array(array=w1760, index (row)=1 ("인덱스 (행)")) -> (deleted portion=w1762:string[])  [unwired: 2 in, 1 out]
        n635 = Unbundle By Name(w1748) -> ("Python 경로"=w1750:path, "지도 모듈 경로"=w1749:path)
        n636 = Build Array(w1762, w1761) -> (w1758:string[][])
        n637 = disable-structure shown="기본" {
          disable-tunnel: [w1765] -> w1751
          frame Enabled {
            w1766 = T11 1 items=["사용자 홈"=0, "사용자 데스크탑"=1, "사용자 문서"=2, "사용자 어플리케이션 데이터"=3, "사용자 환경"=4, "사용자 임시"=5, "퍼블릭 문서"=6, "퍼블릭 어플리케이션 데이터"=7, "퍼블릭 환경"=8, "퍼블릭 캐시"=13, "시스템 코어 라이브러리"=9, "시스템 설치된 라이브러리"=10, "어플리케이션 파일"=11, "부팅 볼륨 루트"=12] ("system directory type")
            # "※ Python 모듈에서 .html 파일의 저장 위치는 데이터 저장 폴더위치와 동일하게 설정한다\n    만약 해당 폴더가 없을 경우 폴더를 생성하여 해당 폴더에 저장한다."
            n638 = call <vilib>:"Get System Directory.vi"("system directory type"=w1766) -> ("system directory"=w1768:path)  [unwired: 10 in]
            n639 = Build Path(base path=w1768, name or relative path="CSV_DATA") -> (appended path=w1772:path)
            n640 = call <vilib>:"Check if File or Folder Exists.vi"("path"=w1772) -> ("error out"=w1771:errorcluster, "file or folder exists?"=w1769:bool, "dup path"=w1770:path)  [unwired: 8 in]
            n641 = case shown="거짓" w1769 {
              tunnel: w1770 -> [w1777 w1779]
              tunnel: w1771 -> [w1776 w1778]
              tunnel: [w1775 w1779] -> w1773
              tunnel: [w1774 w1778] -> _
              frame False {
                n642 = Create Folder(path (use dialog)=w1777, error in=w1776) -> (created path=w1775:path, error out=w1774:errorcluster)  [unwired: 1 in, 1 out]
              }
              frame True {
              }
            }
            n643 = Path To String(path=w1773) -> (string=w1765:string)
          }
        }
        n644 = Delete From Array(array=w1758, index (col)=5 ("비활성화된 인덱스 (열)")) -> (array with subset deleted=w1757:string[][])  [unwired: 2 in, 1 out]
        n645 = Fract/Exp String To Number(string=w1757) -> (number=w1753:dbl[][])  [unwired: 3 in, 1 out]
        n646 = disable-structure shown="기본" {
          disable-tunnel: [w1782] -> w1756
          disable-tunnel: w1753 -> [w1780]
          frame Enabled {
            # "※ 지도 모듈 버튼 작동시 GPS 데이터가 최소 2개이상 들어와야 Python 모듈이 작동된다. 5개의 데이터 중 2개 이상 들어온다면 인덱스 값: 3 \n 에러없이 작동됨에 따라 2개이상 데이터가 없다면 LED 블랭크 작동"
            n647 = for {
              tunnel: w1780 -> [w1786] mode=indexing
              tunnel: [w1784] -> w1782
              tunnel: 0 -> [w1783]
              n648 = Equal To 0?(x=w1786) -> (x = 0?=w1785:bool[])
              n649 = for {
                tunnel: w1785 -> [w1789] mode=indexing
                shift-right: [w1787] -> w1784
                shift-left: w1783 -> [w1788]
                n650 = case shown="참" w1789 {
                  tunnel: w1788 -> [w1790 w1792]
                  tunnel: [w1790 w1791] -> w1787
                  frame False {
                  }
                  frame True {
                    n651 = Increment(x=w1792) -> (x+1=w1791:i32)
                  }
                }
              }
            }
          }
        }
        n652 = call "Reshape_Array_GPS(Subvi).vi"("2차원_GPS_Data"=w1753) -> ("1차원_GPS_Data"=w1752:dbl[])  [unwired: 10 in]
        n653 = Less Or Equal?(x=w1756, y=3) -> (x <= y?=w1754:bool)
        n654 = case shown="참" w1754 {
          tunnel: w1752 -> [_ w1797]
          tunnel: w1751 -> [_ w1796]
          tunnel: w1750 -> [_ w1795]
          tunnel: w1749 -> [_ w1794]
          frame False {
            # "※ 2개이상 없다면 LED 블랭크"
            n655 = property on="지도모듈_LED" class="Bool (엄격한)"("Blinking"=TRUE ("점멸")) -> ()  [unwired: 2 in, 2 out]
          }
          frame True {
            # "※ GPS 데이터가 2개 이상 들어온다면 Python 모듈 실행, 2개이상 있다면 LED 블랭크 F"
            n656 = Open Python Session(python version="3.9" ("Python 버전"), python path=w1795) -> (session out=w1800:refnum<k35>, error out=w1804:errorcluster)  [unwired: 1 in]
            n657 = node(w1800, w1794, "Map" ("함수 이름"), w1804, dbl[] [0.0], w1796, w1797) -> (w1802:refnum<k35>, w1801:errorcluster)  [unwired: 3 in, 2 out]
            n658 = property on="지도모듈_LED" class="Bool (엄격한)"("Blinking"=FALSE ("점멸")) -> ()  [unwired: 2 in, 2 out]
            n659 = Close Python Session(session in=w1802, error in=w1801) -> ()  [unwired: 1 out]
          }
        }
      }
      frame "관리자" {
        # "※ 관리자 버튼 클릭시 탭 컨트롤을 관리자로 변경(Brain_LOOP)"
        n660 = property on="전체메뉴_탭_컨트롤" class="TabCtl (엄격한)"("Value"=enum32{"지도", "데이터 통계", "관리자", "유속 데이터"}."관리자" ("전체메뉴_탭_컨트롤")) -> ()  [unwired: 2 in, 2 out]
      }
      frame "데이터통계" {
        # "※ 데이터통계 버튼 클릭시 탭 컨트롤을 데이터 통계로 변경(Brain_LOOP)"
        n661 = property on="전체메뉴_탭_컨트롤" class="TabCtl (엄격한)"("Value"=enum32{"지도", "데이터 통계", "관리자", "유속 데이터"}."데이터 통계" ("전체메뉴_탭_컨트롤")) -> ()  [unwired: 2 in, 2 out]
      }
      frame "유속 데이터" {
        # "※ 알림 버튼 클릭시 탭 컨트롤을 알림으로 변경(Brain_LOOP)"
        n662 = property on="전체메뉴_탭_컨트롤" class="TabCtl (엄격한)"("Value"=enum32{"지도", "데이터 통계", "관리자", "유속 데이터"}."유속 데이터" ("전체메뉴_탭_컨트롤")) -> ()  [unwired: 2 in, 2 out]
      }
      frame "정지" {
        w1813 = TRUE
        # "※ 정지 버튼 클릭시 탭 컨트롤을 관리자로 변경(Brain_LOOP), 정지 버튼 클릭시 GUI 종료"
        n663 = Enqueue Element(queue=w1816, element=Brain_Loop_CTL."정지", error in (no error)=w1815) -> ()  [unwired: 1 in, 3 out]
        n664 = Quit LabVIEW(quit? (T)=w1813) -> ()
      }
    }
  }
  n665 = Merge Errors(w23, w22, w12, w11) -> (w9:errorcluster)
  n666 = while {
    tunnel: w2 -> [w1830]
    tunnel: w1 -> [w1829]
    tunnel: w17 -> [w1827]
    tunnel: w16 -> [w1826]
    shift-right: [w1819] -> _
    shift-left: string[][] [["", "", "", "", "", ""], ["", "", "", "", "", ""], ["", "", "", "", "", ""], ["", "", "", "", "", "0"], ["", "", "", "", "", ""], ["", "", "", "", "", ""], ["", "", "", "", "", ""], ["", "", "", "", "", "0"], ["", "", "", "", "", ""], ["", "", "", "", "", ""], ["", "", "", "", "", ""], ["", "", "", "", "", ""], ["", "", "", "", "", ""]] -> [w1821]
    tunnel: [errorcluster {"status"=FALSE, "code"=0, "source"=""} ("에러 상수")] -> w10
    stop <- w1828 stop-if-true
    # "Number 데이터 분리 후 리스트 박스 열에 데이터 대체"
    # "3 index: Number"
    n667 = Dequeue Element(queue=w1830, error in (no error)=w1829) -> (queue out=w1825:refnum<queue>, element=w1818:T9, error out=w1824:errorcluster)  [unwired: 1 in, 1 out]
    n668 = Dequeue Element(queue=w1827, error in (no error)=w1826) -> (element=w1820:string[])  [unwired: 1 in, 3 out]
    n669 = case shown="\"정지\"" w1818 {
      tunnel: [_ _ TRUE] -> w1828
      tunnel: w1825 -> [_ w1868 w1873]
      tunnel: w1824 -> [_ w1867 w1872]
      frame "초기화", Default {
      }
      frame "Mqtt_Subscribe" {
        n670 = Enqueue Element(queue=w1868, element=Brain_Loop_CTL."Mqtt_Subscribe", error in (no error)=w1867) -> ()  [unwired: 1 in, 3 out]
      }
      frame "정지" {
        n671 = Flush Queue(queue=w1873, error in (no error)=w1872) -> (queue out=w1870:refnum<queue>, error out=w1871:errorcluster)  [unwired: 1 out]
        n672 = Enqueue Element(queue=w1870, element=Brain_Loop_CTL."정지", error in (no error)=w1871) -> ()  [unwired: 1 in, 3 out]
      }
    }
    n673 = Index Array(array=w1820, index=3 ("인덱스")) -> (element=w1822:string)
    n674 = case shown="\"5\"" w1822 {
      tunnel: w1820 -> [_ w1836 w1843 w1850 w1857 w1864]
      tunnel: w1821 -> [w1831 w1838 w1845 w1852 w1859 w1866]
      tunnel: [w1831 w1832 w1839 w1846 w1853 w1860] -> w1819
      frame "거짓", Default {
      }
      frame "1" {
        # "Number 데이터 분리 후 리스트 박스 열에 데이처 대체"
        n675 = Array Subset(array=w1836, index=0 ("차원 크기"), length=3 ("차원 크기")) -> (w1833:string[])
        n676 = Replace Array Subset(array=w1838, new element=w1833, index (col)=0 ("비활성화된 인덱스 (열)")) -> (w1832:string[][])  [unwired: 1 in]
        n677 = property on="Station_현황_GPS" class="MCListbox (엄격한)"("ItemNames"=w1832) -> ()  [unwired: 2 in, 2 out]
      }
      frame "2" {
        # "Number 데이터 분리 후 리스트 박스 열에 데이처 대체"
        n678 = Array Subset(array=w1843, index=0 ("차원 크기"), length=3 ("차원 크기")) -> (w1840:string[])
        n679 = Replace Array Subset(array=w1845, new element=w1840, index (col)=1 ("비활성화된 인덱스 (열)")) -> (w1839:string[][])  [unwired: 1 in]
        n680 = property on="Station_현황_GPS" class="MCListbox (엄격한)"("ItemNames"=w1839) -> ()  [unwired: 2 in, 2 out]
      }
      frame "3" {
        # "Number 데이터 분리 후 리스트 박스 열에 데이처 대체"
        n681 = Array Subset(array=w1850, index=0 ("차원 크기"), length=3 ("차원 크기")) -> (w1847:string[])
        n682 = Replace Array Subset(array=w1852, new element=w1847, index (col)=2 ("비활성화된 인덱스 (열)")) -> (w1846:string[][])  [unwired: 1 in]
        n683 = property on="Station_현황_GPS" class="MCListbox (엄격한)"("ItemNames"=w1846) -> ()  [unwired: 2 in, 2 out]
      }
      frame "4" {
        # "Number 데이터 분리 후 리스트 박스 열에 데이처 대체"
        n684 = Array Subset(array=w1857, index=0 ("차원 크기"), length=3 ("차원 크기")) -> (w1854:string[])
        n685 = Replace Array Subset(array=w1859, new element=w1854, index (col)=3 ("비활성화된 인덱스 (열)")) -> (w1853:string[][])  [unwired: 1 in]
        n686 = property on="Station_현황_GPS" class="MCListbox (엄격한)"("ItemNames"=w1853) -> ()  [unwired: 2 in, 2 out]
      }
      frame "5" {
        # "Number 데이터 분리 후 리스트 박스 열에 데이처 대체"
        n687 = Array Subset(array=w1864, index=0 ("차원 크기"), length=3 ("차원 크기")) -> (w1861:string[])
        n688 = Replace Array Subset(array=w1866, new element=w1861, index (col)=4 ("비활성화된 인덱스 (열)")) -> (w1860:string[][])  [unwired: 1 in]
        n689 = property on="Station_현황_GPS" class="MCListbox (엄격한)"("ItemNames"=w1860) -> ()  [unwired: 2 in, 2 out]
      }
    }
  }
  n690 = disable-structure shown="비활성화" {
    frame Disabled {
      (unwired) dbl[] [37.5072384, 127.0238756, 37.4172384, 127.1338756, 37.5442384, 127.0448756, 37.4032384, 127.4638756, 37.8055384, 127.7643756]
    }
    frame Enabled {
    }
  }
  n691 = Merge Errors(w9, w10) -> (w8:errorcluster)
  n692 = call <vilib>:"Simple Error Handler.vi"("error in (no error)"=w8) -> ()  [unwired: 4 in, 5 out]
